vi "ControlUI_Main0.vi"(5 "Splash StatusRef":refnum<vi>, 7 "Splash VI Ref":refnum<vi>, 10 "Application":refnum<class "Application.lvclass">, 11 "Main.lvclass":refnum<class "Main.lvclass">) -> ()   [LabVIEW 2019, in "Main.lvclass"]
doc: "Developed by Kevin Thompson\nkevin@thompsonengineering.net\n\nCopyright 2018\nThompson Engineering, LLC"
uses:
  Main.lvclass
  <vilib>/TELLC/SMQ/Add States to Queue using MultiLine String with vData.vi
  Common/DataTypes/TD Async CmdMsg EventData--cluster.ctl
  DataTypes/Public Events--cluster.ctl
  DataTypes/Dependency--cluster.ctl
  DataTypes/Settings--cluster.ctl
  DataTypes/Control UI - AppData--cluster.ctl
  Log_Engine/Log_Engine.lvclass
  DAQ_Engine/DAQ_Engine.lvclass
  Config/Config.lvclass
  Application/Application.lvclass
  Application/DataTypes/AsynMsg_Application--enum.ctl
  Common/DataTypes/TD GetSet ActionSelect--enum.ctl
  Common/Startup/GBL System.vi
  DAQ_Engine/DataTypes/AsynCmd_DAQ_Engine--enum.ctl
  Common/DataTypes/Measurement Config--cluster.ctl
  Common/DataTypes/DAQState--enum.ctl
  Common/DataTypes/LogState--enum.ctl
  Common/DataTypes/TDMSState--enum.ctl
  Common/DataTypes/UpdateControlValue EvData--cluster.ctl
  DataTypes/DataProcessAuxData--cluster.ctl
  Common/DataTypes/DataProcAuxDat--Qref.ctl
  Common/DataTypes/ChannelWaveforms--cluster.ctl
  Common/DataTypes/InverterWaveforms--cluster.ctl
  Common/DataTypes/InverterWaveforms--QRef.ctl
  support/Data Algorithms/subvis/DataTypes/Gain control.ctl
  DataTypes/ProcessingState--enum.ctl
  DataTypes/ProcessingStateChg EvData--cluster.ctl
  DataTypes/InverterInfo--cluster.ctl
  DataTypes/ProcessInitParams--cluster.ctl
  DataTypes/StartProcInitParams--cluster.ctl
  <vilib>/TELLC/Dynamic CVT API/TD Dynamic CVT DVR--ref.ctl
  DataTypes/AsynMsg_Main--enum.ctl
  DataTypes/PrivateAsynEv_Main--enum.ctl
  Common/DataTypes/inverter info v2--cluster.ctl
  Common/DataTypes/inverter gain range--cluster.ctl
  Common/DataTypes/inverter offset range--cluster.ctl
  Common/DataTypes/Inverter database record v2--cluster.ctl
  support/Data Algorithms/subvis/DataTypes/ESR scaling--cluster.ctl
  <userlib>/_OpenG.lib/comparison/comparison.llb/String Changed__ogtk.vi
  <userlib>/_OpenG.lib/error/error.llb/Filter Error Codes (Array)__ogtk.vi
  Common/DataTypes/Acquisition Mode--cluster.ctl
panel:
  out "Next State":string
  in  "Trigger SelectInverter Event":bool
  in  "LeftPanelTab":T1(tab)=enum."Settings"
  out "InvSelLED":bool
  in  "Selected Inverter":string[](array[string])
  in  "SelectInverter":bool
  in  "Inverter List":i32[](listbox)
  in  "Settings.Signal scaling":T2[](array[typedef])
  in  "Samples RMS 9775":u32=3
  in  "Samples RMS 9215":u32=480000
  in  "Data Rate 9215 (S/s)":dbl=1200000.0 format="%#.6p"
  in  "Data Rate 9775(S/s)":dbl=3.0 format="%#.6p"
  out "DAQEnabled":bool=TRUE
  in  "DAQEnDis":bool
  out "LogEnabled":bool
  in  "LogEnDis":bool
  out "TDMSEnabled":bool
  in  "TDMSEnDis":bool
  in  "StopProcessing":bool caption="StopProcess"
  out "Processing":bool=TRUE
  in  "StartProcessing":bool caption="StartProcess"
  in  "UpdateDAQSettings":bool
  in  "Acqusition Mode":T3
  in  "cRIO Error\nReporting Mode":i32(ring) items=["DONTPRINT", "PRINTWARNINGS", "PRINTFATAL", "PRINTALL"]
  in  "MinCurrThreshold":dbl=1.5 caption="Minimum Current\nThreshold (A)" format="%.2f"
  in  "NumPF RdsToAvg":i32=2 caption="Number PF\nReads to Avg"
  in  "ESR alarm threshhold (%)":dbl=200.0
  in  "# readings to average":i32=40
  out "DP AuxData Size":i32
  out "InvWfmsQ DT size":i32
  in  "Inverter ID":string
  in  "toggle scrollbars":bool
  in  "toggle MainTabDbgPg":bool
  out "voltage fb":dbl caption="Voltage" format="%.3f"
  out "Current fb":dbl caption="Current" format="%.3f"
  out "Motor SP":dbl caption="Computed Motor\nPos Chg (in)" format="%.3f"
  out "In Range?":bool
  out "AVC Lockout":bool=TRUE
  out "Volts and Current Chart":T4(graph)
  out "VoltageError":dbl caption="Voltage Error" format="%.3f"
  in  "Launch_UI":bool caption="Launch UI"
  in  "Launch_UI 2":bool caption="Launch UI 2"
  in  "Launch_UI 3":bool caption="Launch UI 3"
  out "Current SP":dbl format="%.3f"
  in  "GraphEnable":bool
  out "Vsp_Sum":dbl format="%.2f"
  out "TotalVgain":dbl caption="Total Ctlr\nVgain" format="%.3f"
  out "DAQ Running":bool=TRUE
  out "MeasSet":T5={"Data Rate 9775"=3.0, "Data Rate 9215"=1200000.0, "Samples RMS 9215"=480000, "Samples RMS 9775"=3}
  out "DAQError":bool caption="DAQ Error"
  in  "SystemError":bool
  out "Sel_PowerFactor_Data":bool=TRUE
  in  "Show_PowerFactor_Data":bool
  out "Sel_TimeSeries_Data":bool
  in  "Show_TimeSeries_Data":bool
  out "Sel_ESR_Data":bool
  in  "Show_ESR_Data":bool
  in  "MainPanelTab":T6(tab)=enum."PowerFactorData"
  out "Max ESR":dbl format="%_4e"
  out "Inverter State":string
  out "Equivalent Series Resistance (ESR)":T7(graph)
  in  "StoreESR BLine":bool
  in  "UseSavedESR BLine":bool
  in  "set alarm":bool
  in  "reset averaging":bool
  in  "reset alarm":bool
  out "Inverter ESR status":bool
  out "Raw  ESR":dbl format="%.3e"
  out "Scaled & avgd ESR":dbl format="%_4e"
  in  "ESR scaling":T8[](array[typedef])
  out "Iout 60Hz":waveform(dbl)[](graph)
  out "Iout ripple":waveform(dbl)[](graph)
  out "Iin ripple":waveform(dbl)[](graph)
  out "DUT4 I-V":waveform(dbl)[](graph) caption="DUT 4"
  out "phase3 power data":T9 caption="Phase 1" {"Vout (RMS)" format="%0.2f"; "Iout (RMS)" format="%0.2f"; "PF" format="%.3g"}
  out "phase2 power data":T9 caption="Phase 1" {"Vout (RMS)" format="%0.2f"; "Iout (RMS)" format="%0.2f"; "PF" format="%.3g"}
  out "DUT3 I-V":waveform(dbl)[](graph) caption="DUT 3"
  out "DUT2 I-V":waveform(dbl)[](graph) caption="DUT 2"
  out "DUT1 I-V":waveform(dbl)[](graph) caption="DUT 1"
  out "phase1 power data":T9 caption="Phase 1" {"Vout (RMS)" format="%0.2f"; "Iout (RMS)" format="%0.2f"; "PF" format="%.3g"}
  in  "Dummy Vrms":dbl format="%.2g"
  in  "UseDummyVrms":bool
  out "phase4 power data":T9 caption="Phase 1" {"Vout (RMS)" format="%0.2f"; "Iout (RMS)" format="%0.2f"; "PF" format="%.3g"}
  in  "Page2Pg_button":bool
  in  "SettingsPg_button":bool
  in  "DataPg_button":bool
  in  "ConfigPg_button":bool
  in  "Exit":bool
  in  "TitleBar AppVerText":string="v2.0.2 build-003"
  in  "TitleBar Text":string="INVERTER   HEALTH   SCANNER   SYSTEM"
  in  "TitleBar":bool
  in  "StatusMsg":string caption="Status"
  in  "process sync":refnum<notifier>
  # "click to reset"
  # "UNUSED CONTROLS"
  # "Run Time Data Panel"
  # "Inverter Selection"
  # "right-click to open table editor"
  # "Configuration Panel"
  # "Settings Panel"
  # "cRIO  Settings"
  # "ESR Data"
  # "Time Series Data"
  # "DUT 1"
  # "DUT 2"
  # "DUT 3"
  # "DUT 4"
  # "Power Factor Data - Phase Current and Voltage"
  # "DUT 3"
  # "DUT 2"
  # "DUT 1"
  # "Current (A)"
  # "Voltage (V)"
  # "DUT 4"
  # "Debug Page"
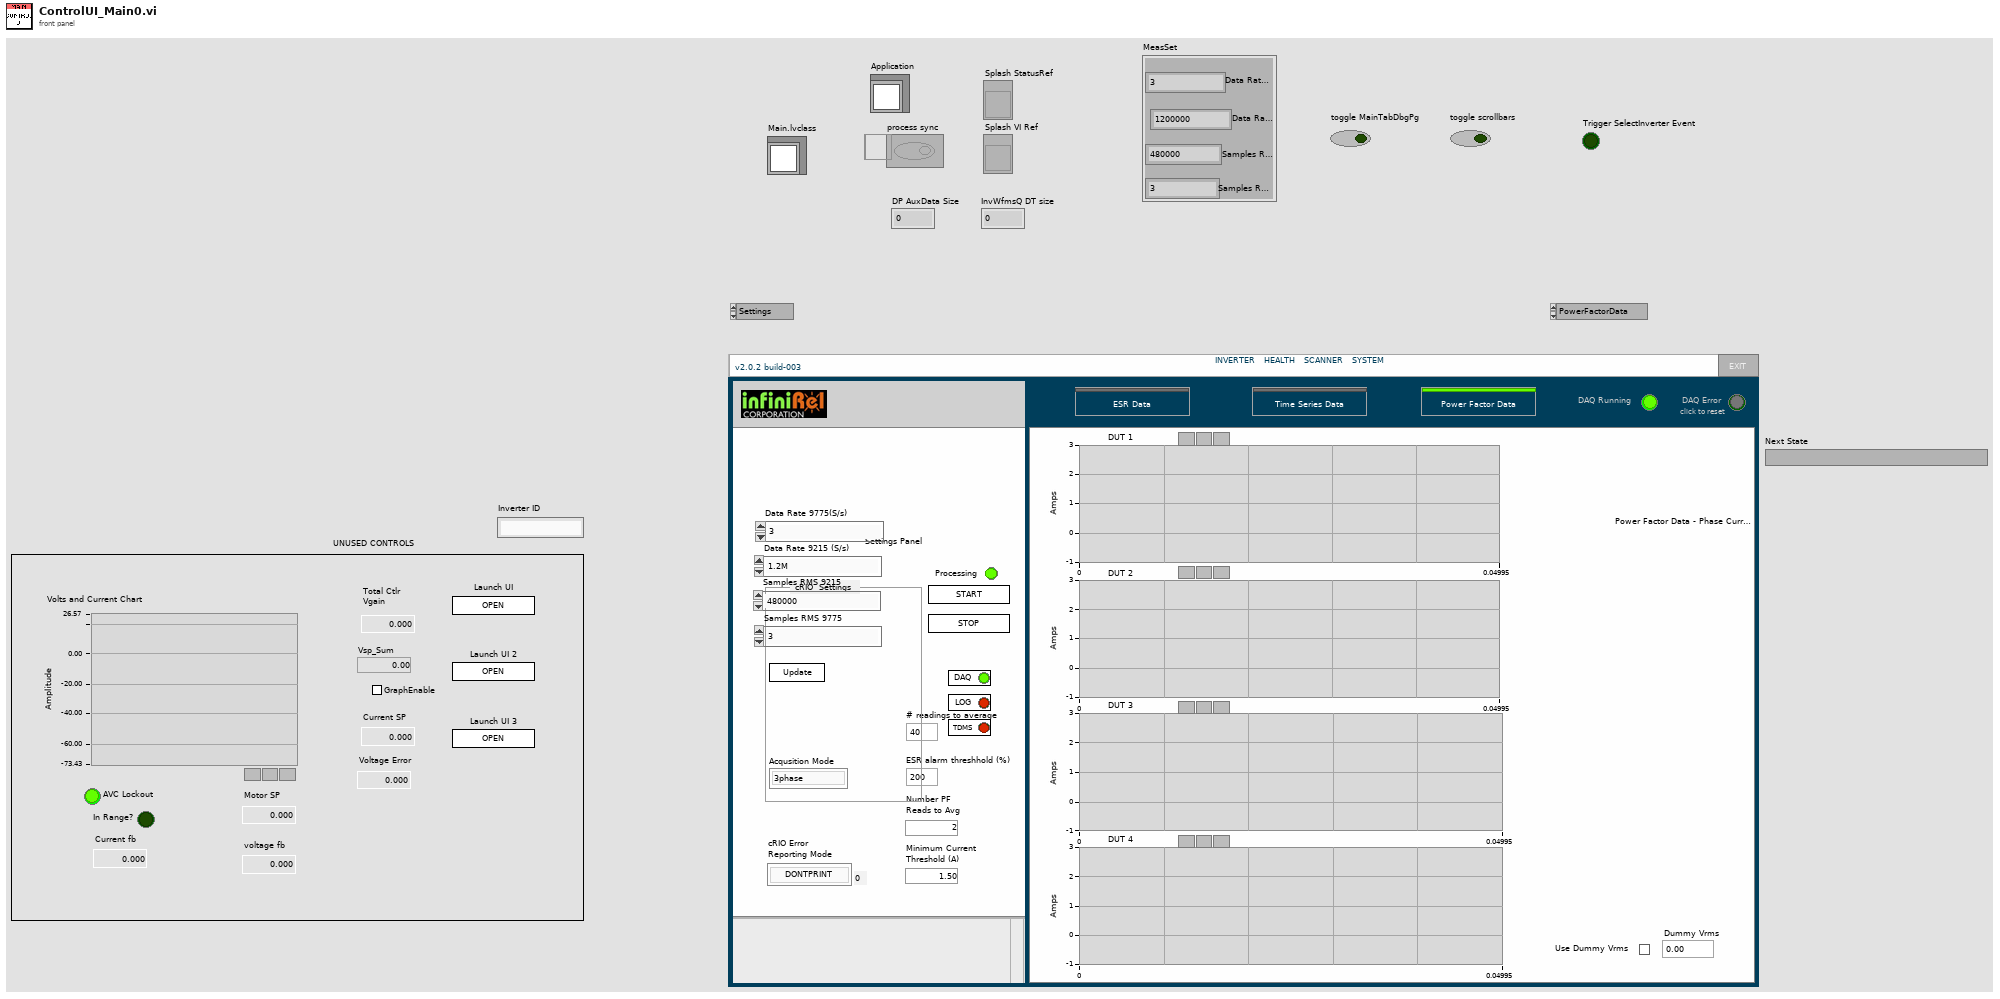
[diagram p1: front panel]
types:
  T1 = enum32{"Data", "InverterSel", "Config", "Settings"}
  T2 = typedef "Main.lvclass/Gain control.ctl" = cluster{"Iin ripple gain":dbl, "Iout ripple gain":dbl, "Iout 60Hz gain ":dbl, "Vout 60Hz gain ":dbl, "Iin ripple offest":dbl, "Iout ripple offset":dbl, "Iout 60Hz offset":dbl, "Vout 60Hz offset":dbl}
  T3 = typedef "Acquisition Mode--cluster.ctl" = enum16{"3phase", "Single"}
  T4 = cluster{"VoltageDyn":dbl, "CurrentDyn":dbl, "MotorV SP":dbl}
  T5 = typedef "Measurement Config--cluster.ctl" = cluster{"Data Rate 9775":dbl, "Data Rate 9215":dbl, "Samples RMS 9215":u32, "Samples RMS 9775":u32}
  T6 = enum32{"ESRData", "TimeSeriesData", "PowerFactorData", "DebugPage"}
  T7 = cluster{"ESR Baseline":dbl, "Alarm threshhold (%)":dbl, "Avg value":dbl}[]
  T8 = typedef "Main.lvclass/ESR scaling--cluster.ctl" = cluster{"Gain":dbl, "Offset":dbl}
  T9 = cluster{"PF":dbl, "Iout (RMS)":dbl, "Vout (RMS) ":dbl, "Power (W)":dbl}
  T10 = typedef "Main.lvclass/ProcessingState--enum.ctl" = enum16{"Idle", "Starting", "Running", "Done", "Error"}
  T11 = typedef "TD GetSet ActionSelect--enum.ctl" = enum16{"Init", "Get", "Set"}
  T12 = typedef "Main.lvclass/Control UI - AppData--cluster.ctl" = cluster{"Core":cluster{"Current VI Reference":refnum<vi>, "Close Panel on Exit?":bool}, "SMQ":refnum<queue>, "Initialized?":bool, "Self Reference":refnum<class "Main.lvclass">, "Simulation?":bool, "process sync":refnum<notifier>, "vData":variant, "Settings":T13, "Dependency":T14, "Public Events":T15, "Splash StatusRef":refnum<vi>, "Splash VI Ref":refnum<vi>, "RunTimeSystem?":bool, "StatusMsg Ref":refnum<vi>, "AppTerminateEv":refnum<user-event>, "MenuRef":refnum<k9>, "DAQEnabled":bool, "LoggingEnabled":bool, "TDMS Enabled":bool, "Application":refnum<class "Application.lvclass">, "InvWfmsQ-DT":T16, "DPAuxDataQ":T17, "ProcessingState":T10, "DisplayLoopInterval":u32, "MenuBarShown?":bool, "InverterNames[]":string[], "InverterLUT Dict":T18}
  T13 = typedef "Main.lvclass/Settings--cluster.ctl" = cluster{"Simulation":bool, "Signal scaling":T2[], "ESR scaling":T8[], "num readings to average":i32[], "ESR alarm threshhold (%)":i32[], "UseDummyVrms":bool, "Dummy Vrms":dbl, "Inverter Database File":path, "default Inverter (name)":string[]}
  T14 = typedef "Main.lvclass/Dependency--cluster.ctl" = cluster{"Config":refnum<class "Config.lvclass">, "DAQ":refnum<class "DAQ_Engine.lvclass">, "Log_Engine":refnum<class "Log_Engine.lvclass">}
  T15 = typedef "Main.lvclass/Public Events--cluster.ctl" = cluster{"Main.AsyncCmd Event":refnum<user-event>, "Main.AsyncMsg Event":refnum<user-event>, "stop process":refnum<user-event>, "UpdateControlValue Ev":refnum<user-event>, "ProcessingStateChg Ev":refnum<user-event>}
  T16 = typedef "InverterWaveforms--QRef.ctl" = refnum<queue>
  T17 = typedef "DataProcAuxDat--Qref.ctl" = refnum<queue>
  T18 = typedef "TD Dynamic CVT DVR--ref.ctl" = refnum<data-value>
  T19 = cluster{"AvgPF":dbl, "IoutRMS_A":dbl, "VoutRMS_V":dbl, "Power_W":dbl}
  T20 = typedef "DataProcessAuxData--cluster.ctl" = cluster{"Time Stamp":timestamp, "Raw ESR sum":dbl, "Inv 1 ON?":bool, "Average scaled ESR sum":dbl, "Inv 1 over threshold?":bool, "Inv 1 ESR":cluster{"ESR Baseline":dbl, "Alarm threshhold (%)":dbl, "Avg value":dbl}, "Max ESR":dbl}
  T21 = cluster{"ESR Baseline":dbl, "Alarm threshhold (%)":dbl, "Avg value":dbl}
  T22 = typedef "InverterWaveforms--cluster.ctl" = T23[]
  T23 = typedef "ChannelWaveforms--cluster.ctl" = cluster{"Iin ripple ":waveform(dbl), "Iout ripple ":waveform(dbl), "Iout 60Hz":waveform(dbl), "Vout 60Hz":waveform(dbl)}
  T24 = typedef "DAQ_Engine.lvclass/AsynCmd_DAQ_Engine--enum.ctl" = enum16{"DAQ.EnableDAQ", "DAQ.ClearDAQError", "DAQ.SetMeasConfig", "DAQ.SetAcqMode", "DAQ.SetErrorReporting"}
  T25 = typedef "Main.lvclass/StartProcInitParams--cluster.ctl" = cluster{"InverterInfo":T26, "ProcessInitParams":T27}
  T26 = typedef "InverterInfo--cluster.ctl" = cluster{"Inverter ID":string}
  T27 = typedef "Main.lvclass/ProcessInitParams--cluster.ctl" = cluster{"MinCurrThreshold":dbl, "NumPF RdsToAvg":i32, "ESR alarm threshhold (%)":dbl, "# readings to average":i32}
  T28 = typedef "Main.lvclass/PrivateAsynEv_Main--enum.ctl" = enum16{"PrivMain.UpdateMeasSettings", "PrivMain.UpdateAcqMode", "PrivMain.UpdateDAQState", "PrivMain.UpdateLogState", "PrivMain.UpdateTDMSState", "PrivMain.UpdateProcessingState", "PrivMain.Stop&Terminate", "PrivMain.CurrInverterUpdated", "PrivMain.UpdateStoreUseESRBaseline", "PrivMain.SetUnsetAlarm&ESRBLine", "PrivMain.ResetAveraging"}
  T29 = typedef "Main.lvclass/AsynMsg_Main--enum.ctl" = enum16{"Main.CurrInverterUpdated"}
  T30 = typedef "DAQState--enum.ctl" = enum16{"Unknown", "Stopped", "Running", "Error"}
  T31 = cluster{"VoltageDyn":dbl, "CurrentDyn":dbl, "MotorV SP":dbl}[]
  T32 = enum32{"invalid app kind", "Development System", "Run Time System", "Student Edition", "Embedded LabVIEW", "Evaluation", "Custom"}
  T33 = typedef "Application.lvclass/AsynMsg_Application--enum.ctl" = enum16{"Application.AppClassReference"}
  T34 = enum16{"Left Button", "Center Button", "Right Button", "Window Close"}
  T35 = enum32{"Invalid", "Standard", "Closed", "Hidden", "Minimized", "Maximized"}
  T36 = enum32{"Invalid", "Default", "Floating", "Floating/Auto-Hide", "Modal"}
  T37 = typedef "Inverter database record v2--cluster.ctl" = cluster{"name":string, "last updated":timestamp, "type":string, "inverter Info":T38, "gain range":T39, "offset range":T40, "gain actual":dbl, "offset actual":dbl, "power level":dbl, "minimum current":dbl, "resistance single phase":dbl, "resistance 3 phase":dbl, "set flag":u16}
  T38 = typedef "inverter info v2--cluster.ctl" = cluster{"manufacturer":string, "model":string, "product":string, "serial":string, "power class":string, "year manf":string}
  T39 = typedef "inverter gain range--cluster.ctl" = cluster{"gain max":dbl, "gain min":dbl, "gain increment":dbl}
  T40 = typedef "inverter offset range--cluster.ctl" = cluster{"offset max":dbl, "offset min":dbl, "offset increment":dbl}
  T41 = typedef "Application.lvclass/AVC2_TouchScreen_MainUI - AppData--cluster.ctl" = cluster{"Core":cluster{"Current VI Reference":refnum<vi>, "Close Panel on Exit?":bool}, "SMQ":refnum<queue>, "Initialized?":bool, "Public Events":T42, "Dependency":T43, "MenuRef":refnum<k9>, "RuntimeSystem?":bool, "StatusMsg Ref":refnum<vi>, "PrevSeqFolder":path, "SeqRunning?":bool, "SeqExecStatus":T44, "SeqAborted?":bool, "LoadSeqStatus":T45, "Session Settings":T46, "SessionSettings Set?":bool, "DAQEnabled":bool, "LoggingEnabled":bool, "TDMS Enabled":bool, "Logger State Data":T47, "Splash VI Ref":refnum<vi>, "Splash StatusRef":refnum<vi>, "Motor_LA CtrlUI VI Ref":refnum<vi>, "Dflt_Motor_LA Vel":dbl, "Motor_TT CtrlUI VI Ref":refnum<vi>, "Dflt_Motor_TT Vel":dbl, "App Settings":T49, "ExpSubsysRsp":string, "ExpSubsysRspTime":dbl, "Motor_Osc CtrlUI VI Ref":refnum<vi>, "Dflt_Motor_Osc Vel":dbl, "RGrph":refnum<queue>, "Private Events":T59, "WeldGrph":refnum<queue>, "SeqStartTime (s)":dbl, "XYGraphPlotData":T60, "Seq WeldProfileData":cluster{"Time (s)":dbl[], "WeldCurrent":dbl[]}, "Rect":T61, "MenuBarShown?":bool, "Disable Oscillator Motor":bool, "PurgeTimerExp":dbl, "vData":variant, "WELD COUNT":i32}
  T42 = typedef "Application.lvclass/Public Events--cluster.ctl" = cluster{"Application.AsyncCmd Event":refnum<user-event>, "Application.AsyncMsg Event":refnum<user-event>, "stop process":refnum<user-event>, "Application.ControlStateChg Event":refnum<user-event>, "Application.RadialGraph Event":refnum<user-event>}
  T43 = typedef "Application.lvclass/Dependency--cluster.ctl" = cluster{"Config":refnum<class "Config.lvclass">, "DAQ":refnum<class "DAQ.lvclass">, "Sequencer":refnum<class "Sequencer.lvclass">, "LogEngine":refnum<class "LogEngine.lvclass">, "ErrorHandler":refnum<class "ErrorHandler.lvclass">, "DataQueues":refnum<class "DataQueues.lvclass">, "Motion":refnum<class "Motion.lvclass">, "PID_Ctlr":refnum<class "PID_Ctlr.lvclass">, "Welder":refnum<class "Welder.lvclass">}
  T44 = typedef "Sequencer.lvclass/SeqExecStatus--enum.ctl" = enum16{"Unknown", "Idle", "Running", "Aborted"}
  T45 = typedef "Sequencer.lvclass/LoadSeqStatus--enum.ctl" = enum16{"Unknown", "InProgress", "Loaded", "Failed"}
  T46 = typedef "SessionSettings--cluster.ctl" = cluster{"Job_ID":string, "Operator_ID":string, "Station_ID":string, "Job_Description":string}
  T47 = typedef "LogEngine.lvclass/TD Logger State Data--cluster.ctl" = cluster{"Logger State":T48, "TDMS Logging State":T48, "LogFile path":path, "TDMS File path":path, "vData":variant}
  T48 = typedef "LogEngine.lvclass/TD Logger State--enum.ctl" = enum16{"Unknown", "Logging", "NotLogging", "Error"}
  T49 = typedef "Application.lvclass/Settings--cluster.ctl" = cluster{"Placeholder":bool, "ProfilePlotScaleFactor":dbl, "ConversionFactors":T50, "SystemDefaults":T51, "TimingIntervals":T52, "AO IONames":T53, "DO IONames":T54, "UI Labels":T55, "AI IONames":T56, "DI IONames":T57, "TurntableType":T58, "Torch IncrButton displ (in)":dbl, "preventSimulatedEMOAbort":bool}
  T50 = typedef "Application.lvclass/ConversionFactors--cluster.ctl" = cluster{"WeldCurrentSP I/V":dbl, "Turntable RPM/V":dbl, "VoltageDynFB V/V":dbl, "CurrentDynFB I/V":dbl}
  T51 = typedef "Application.lvclass/SystemDefaults--cluster.ctl" = cluster{"AVCLockout":dbl, "TurntableJog":dbl, "ProfilePlotScaleFactor":dbl, "DefaultSeqFile":string, "defaultVelocitySP":dbl}
  T52 = typedef "Application.lvclass/Timing Intervals--cluster.ctl" = cluster{"DAQDisplay Interval":i32, "DAQRd&MtrSP Interval":u32, "WriteLogFile Interval":u32, "SeqHoldLoop Interval":u32, "SeqRampLoop Interval":u32, "ArcEnRelayToggle Interval":u32}
  T53 = typedef "AO IONames--cluster.ctl" = cluster{"Weld Current":string, "Turntable Speed":string, "Turntable Jog":string}
  T54 = typedef "DO IONames--cluster.ctl" = cluster{"Arc Enable Relay":string, "AVC Lockout Relay":string, "Turntable Enable Relay":string, "Turntable Jog Switch":string}
  T55 = typedef "UI Controls-Indicators Labels--cluster.ctl" = cluster{"SeqRunning":string, "Process Complete":string, "AVC Lockout":string, "Step Comment":string, "StepCntDn":string, "SeqList":string, "Current SP":string, "VspOffset":string, "WeldCurrentWfmChart":string, "Turntable En (Anlg)":string}
  T56 = typedef "AI IONames--cluster.ctl" = cluster{"AI TaskName":string, "VoltageDyn":string, "CurrentDyn":string}
  T57 = typedef "DI IONames--cluster.ctl" = cluster{"DI TaskName":string, "EMO_Signal":string}
  T58 = typedef "TurntableType--enum.ctl" = enum16{"SmartMotor", "Analog"}
  T59 = typedef "Application.lvclass/Private Events--cluster.ctl" = cluster{"Private.AsyncCmd Event":refnum<user-event>, "Private.AsyncMsg Event":refnum<user-event>}
  T60 = typedef "Application.lvclass/WeldCurrent_GraphPlotData--cluster.ctl" = cluster{"Timeoffset(s)":dbl[], "WeldCurrent[]":dbl[]}
  T61 = typedef "LVRectTypeDef.ctl" = cluster{"Left":i16, "Top":i16, "Right":i16, "Bottom":i16}
  T62 = typedef "Main.lvclass/AsynCmd_Main--enum.ctl" = enum16{"Main.StartProcessing", "Main.StopProcessing", "Main.RefreshInverterList"}
  T63 = typedef "DAQ_Engine.lvclass/DAQStateEvData--cluster.ctl" = cluster{"DAQState":T30, "vData":variant}
  T64 = typedef "LogState--enum.ctl" = enum16{"Unknown", "Stopped", "Running", "Error"}
  T65 = typedef "Log_Engine.lvclass/LogStateEvData--cluster.ctl" = cluster{"LogState":T64, "vData":variant}
  T66 = typedef "TDMSState--enum.ctl" = enum16{"Unknown", "Stopped", "Running", "Error"}
  T67 = typedef "Log_Engine.lvclass/TDMSStateEvData--cluster.ctl" = cluster{"TDMSState":T66, "vData":variant}
  T68 = typedef "DAQ_Engine.lvclass/Public Events--cluster.ctl" = cluster{"DAQ_Engine.AsyncCmd Event":refnum<user-event>, "DAQ_Engine.AsyncMsg Event":refnum<user-event>, "stop process":refnum<user-event>, "DAQ_Engine.DAQStateChg Ev":refnum<user-event>, "DAQ_Engine.MeasSettingsChg Ev":refnum<user-event>, "DAQ_Engine.AcqModeChg Ev":refnum<user-event>}
  T69 = typedef "Log_Engine.lvclass/Public Events--cluster.ctl" = cluster{"Log_Engine.AsyncCmd Event":refnum<user-event>, "Log_Engine.AsyncMsg Event":refnum<user-event>, "stop process":refnum<user-event>, "Log_Engine.LogStateChg Ev":refnum<user-event>, "Log_Engine.TDMSStateChg Ev":refnum<user-event>}
  T70 = cluster{"Current VI Reference":refnum<vi>, "Close Panel on Exit?":bool}
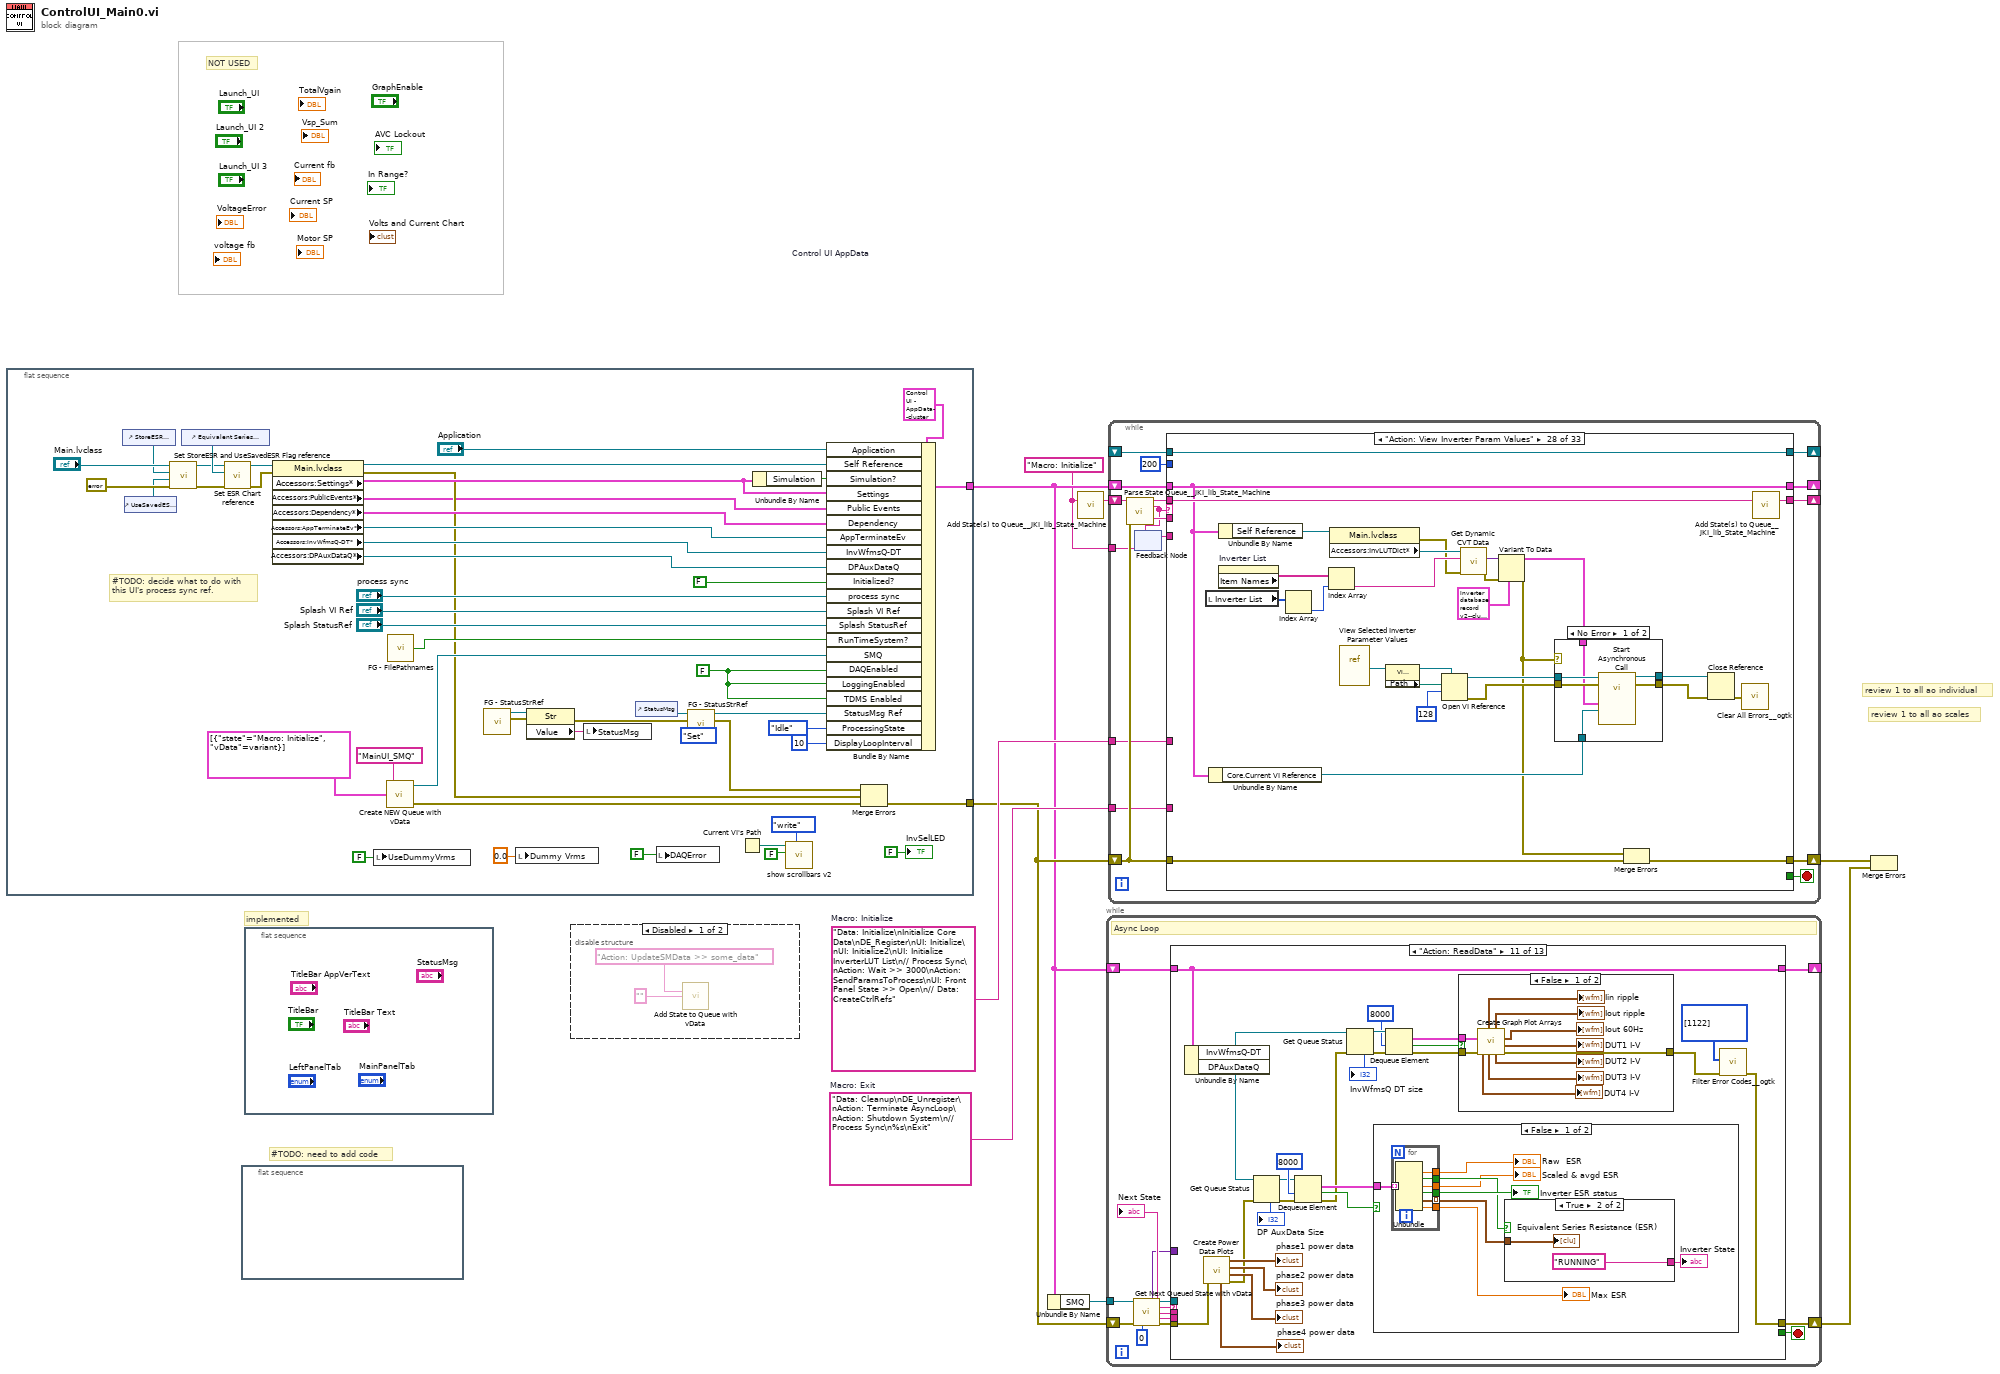
[diagram p0: block diagram]
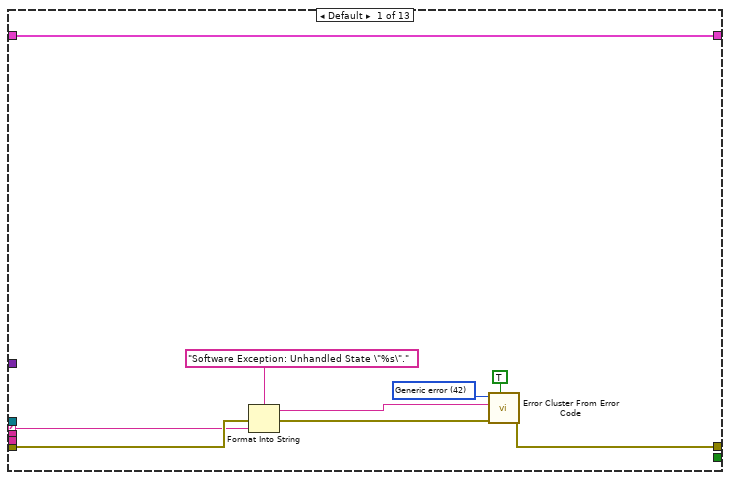
[diagram p3: hidden frame]
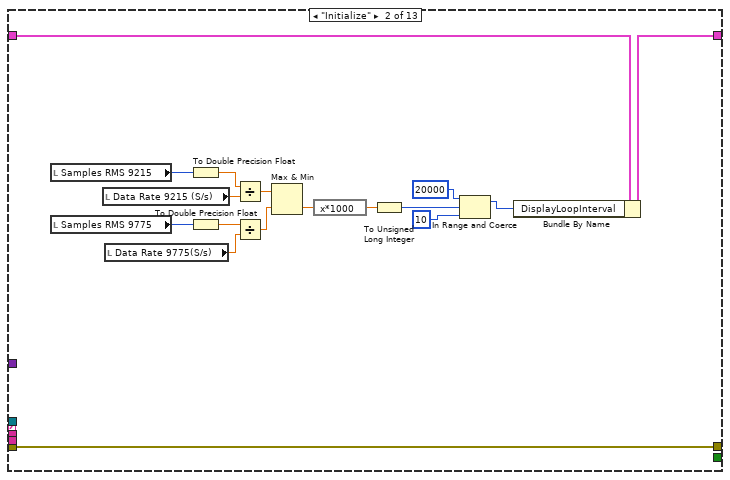
[diagram p4: hidden frame]
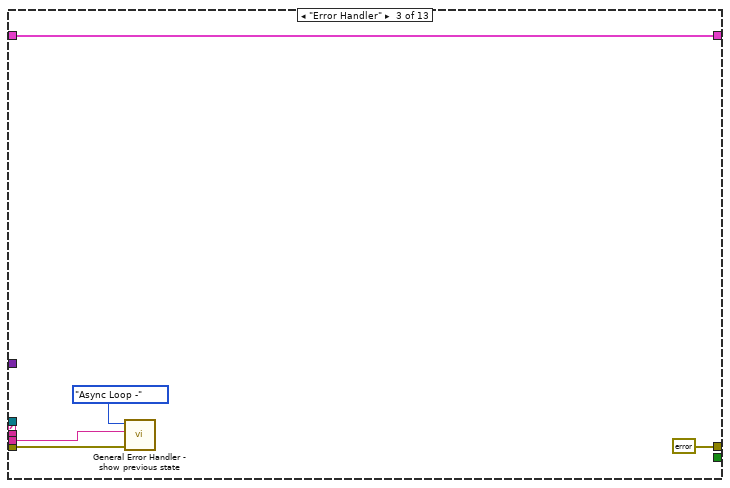
[diagram p5: hidden frame]
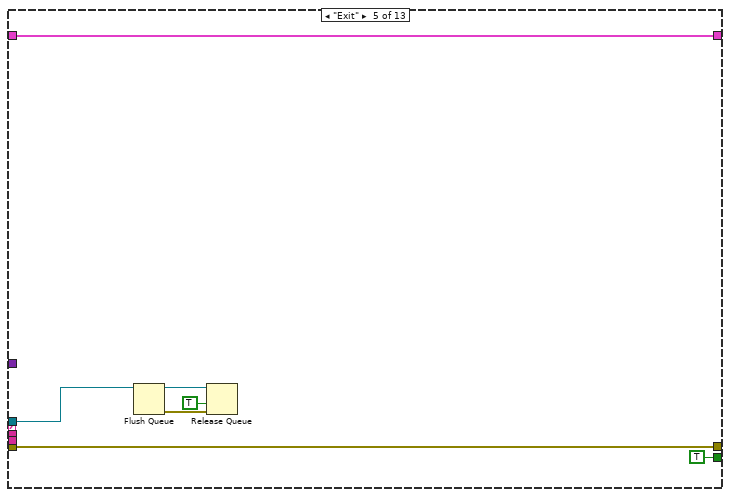
[diagram p7: hidden frame]
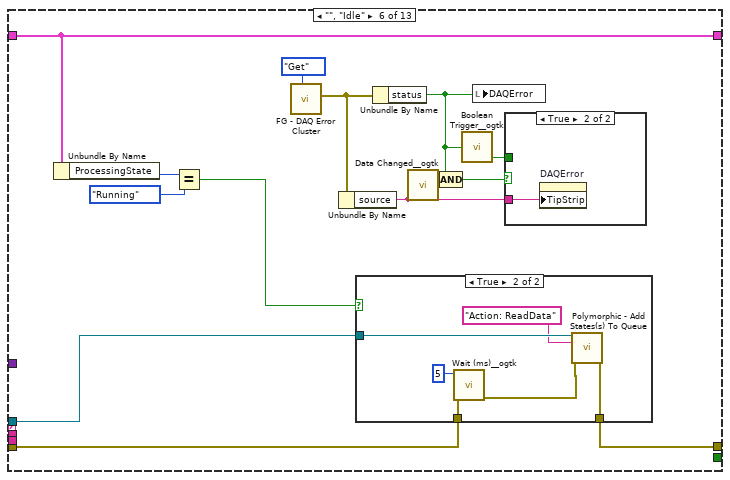
[diagram p8: hidden frame]
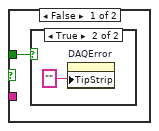
[diagram p9: hidden frame]
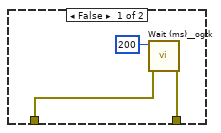
[diagram p11: hidden frame]
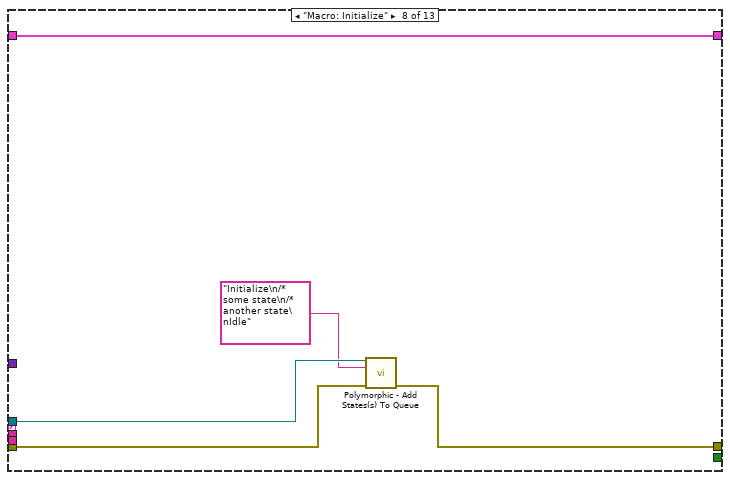
[diagram p13: hidden frame]
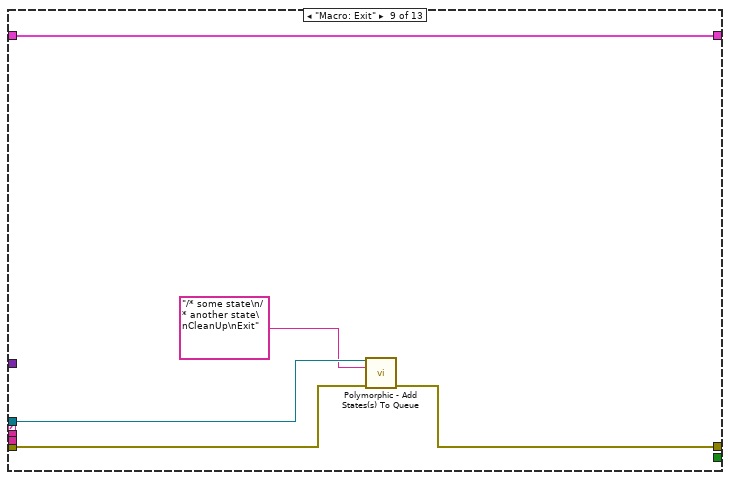
[diagram p14: hidden frame]
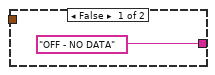
[diagram p16: hidden frame]
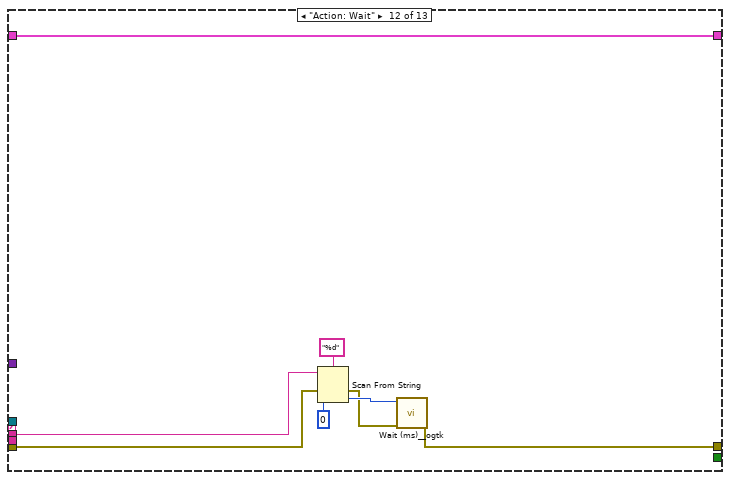
[diagram p19: hidden frame]
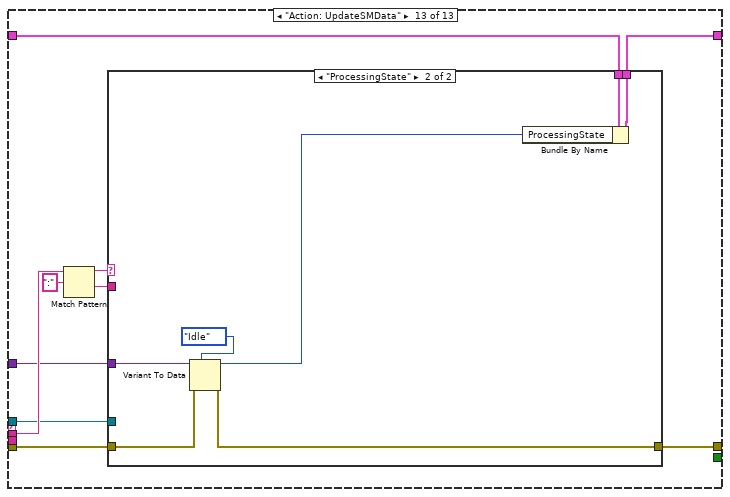
[diagram p20: hidden frame]
diagram:
  w7 = "Data: Cleanup\nDE_Unregister\nAction: Terminate AsyncLoop\nAction: Shutdown System\n// Process Sync\n%s\nExit"  # Macro: Exit
  w8 = "Data: Initialize\nInitialize Core Data\nDE_Register\nUI: Initialize\nUI: Initialize2\nUI: Initialize InverterLUT List\n// Process Sync\nAction: Wait >> 3000\nAction: SendParamsToProcess\nUI: Front Panel State >> Open\n// Data: CreateCtrlRefs"  # Macro: Initialize
  w1 = "Macro: Initialize"
  # "review 1 to all ao scales"
  # "review 1 to all ao individual"
  # "implemented"
  # "#TODO: need to add code"
  # "NOT USED"
  n1 = flat-sequence {
    tunnel: [w58] -> w4
    tunnel: [w43] -> w6
    frame #0 {
      w29 = FALSE
      w50 = T12 {"Core"={"Current VI Reference"=refnum, "Close Panel on Exit?"=FALSE}, "SMQ"=refnum, "Initialized?"=FALSE, "Self Reference"=refnum, "Simulation?"=FALSE, "process sync"=refnum, "vData"=variant, "Settings"={"Simulation"=FALSE, "Signal scaling"=[], "ESR scaling"=[], "num readings to average"=[], "ESR alarm threshhold (%)"=[], "UseDummyVrms"=FALSE, "Dummy Vrms"=0.0, "Inverter Database File"=path "", "default Inverter (name)"=[]}, "Dependency"={"Config"=refnum, "DAQ"=refnum, "Log_Engine"=refnum}, "Public Events"={"Main.AsyncCmd Event"=refnum, "Main.AsyncMsg Event"=refnum, "stop process"=refnum, "UpdateControlValue Ev"=refnum, "ProcessingStateChg Ev"=refnum}, "Splash StatusRef"=refnum, "Splash VI Ref"=refnum, "RunTimeSystem?"=FALSE, "StatusMsg Ref"=refnum, "AppTerminateEv"=refnum, "MenuRef"=refnum, "DAQEnabled"=FALSE, "LoggingEnabled"=FALSE, "TDMS Enabled"=FALSE, "Application"=refnum, "InvWfmsQ-DT"=refnum, "DPAuxDataQ"=refnum, "ProcessingState"=enum."Idle", "DisplayLoopInterval"=0, "MenuBarShown?"=FALSE, "InverterNames[]"=[], "InverterLUT Dict"=refnum}  # Control UI AppData
      # "#TODO: decide what to do with\nthis UI's process sync ref."
      n2 = control-ref of="StoreESR BLine"() -> (w10:refnum<vi>)
      n3 = control-ref of="UseSavedESR BLine"() -> (w11:refnum<vi>)
      n4 = call "Set StoreESR and UseSavedESR Flag reference.vi"("error in (no error)"=errorcluster {"status"=FALSE, "code"=0, "source"=""} ("error constant"), "UseSavedESR BLine Ref"=w11, "StoreESR BLine Ref"=w10, "Main in"="Main.lvclass") -> ("error out"=w14:errorcluster, "Main out"=w15:refnum<class "Main.lvclass">)  [unwired: 6 in]
      n5 = control-ref of="Equivalent Series Resistance (ESR)"() -> (w17:refnum<vi>)
      n6 = call "Set ESR Chart reference.vi"("error in (no error)"=w14, "ESR Chart Ref"=w17, "Main in"=w15) -> ("error out"=w12:errorcluster, "Main out"=w18:refnum<class "Main.lvclass">)  [unwired: 7 in]
      n7 = property class="Main.lvclass"(reference=w18, error in=w12) -> (reference out=w21:refnum<class "Main.lvclass">, error out=w22:errorcluster, "Accessors:Settings*"=w52:T13, "Accessors:PublicEvents*"=w20:T15, "Accessors:Dependency*"=w54:T14, "Accessors:AppTerminateEv*"=w49:refnum<user-event>, "Accessors:InvWfmsQ-DT*"=w28:T16, "Accessors:DPAuxDataQ*"=w27:T17)
      n8 = local write "UseDummyVrms"(FALSE ("UseDummyVrms")) -> ()
      n9 = call <vilib>:"Create NEW Queue with vData.vi"("Initial States"=cluster{"state":string, "vData":variant}[] [{"state"="Macro: Initialize", "vData"=variant}], "Name (SMQ)"="MainUI_SMQ") -> ("error out"=w44:errorcluster, "queue out"=w48:refnum<queue>)  [unwired: 2 in]
      n10 = call "FG - FilePathnames.vi"() -> ("RunTimeSys?"=w45:bool)  [unwired: 4 in, 1 out]
      n11 = call "FG - StatusStrRef.vi"() -> ("StatusStr Ref out"=w42:refnum<vi>, "error out"=w41:errorcluster)  [unwired: 9 in]
      n12 = local write "Dummy Vrms"(0.0 ("Dummy Vrms")) -> ()
      n13 = property class="Str"(reference=w42, error in=w41) -> (error out=w40:errorcluster, "Value"=w39:string)  [unwired: 1 out]
      n14 = local write "StatusMsg"(w39) -> ()
      n15 = control-ref of="StatusMsg"() -> (w38:refnum<vi>)
      n16 = local write "DAQError"(FALSE ("SystemError")) -> ()
      n17 = call "FG - StatusStrRef.vi"("StatusStr Ref in"=w38, "error in (no error)"=w40, "action (Get)"=TD_GetSet_ActionSelect--enum."Set") -> ("StatusStr Ref out"=w36:refnum<vi>, "error out"=w35:errorcluster)  [unwired: 6 in]
      n18 = Current VI's Path() -> (path=w34:path)
      n19 = Unbundle By Name(w52) -> ("Simulation"=w53:bool)
      n20 = call <vilib>:"show scrollbars v2.vi"("mode (read)"=enum16{"read", "write", "toggle"}."write", "ShowScrollbars?"=FALSE, "vi path"=w34) -> ()  [unwired: 4 in, 2 out]
      n21 = Bundle By Name(cluster=w50, "Application"="Application", "Self Reference"=w21, "Simulation?"=w53, "Settings"=w52, "Public Events"=w20, "Dependency"=w54, "AppTerminateEv"=w49, "InvWfmsQ-DT"=w28, "DPAuxDataQ"=w27, "Initialized?"=FALSE, "process sync"="process sync", "Splash VI Ref"="Splash VI Ref", "Splash StatusRef"="Splash StatusRef", "RunTimeSystem?"=w45, "SMQ"=w48, "DAQEnabled"=w29, "LoggingEnabled"=w29, "TDMS Enabled"=w29, "StatusMsg Ref"=w36, "ProcessingState"=ProcessingState--enum."Idle", "DisplayLoopInterval"=u32 10) -> (w58:T12)
      n22 = Merge Errors(w35, w22, w44) -> (w43:errorcluster)
      "InvSelLED" <- FALSE ("InvSelLED")
    }
  }
  n23 = flat-sequence {
    frame #0 {
    }
  }
  n24 = flat-sequence {
    frame #0 {
    }
  }
  n25 = disable-structure shown="Disabled" {
    frame Disabled {
      n26 = call <vilib>:"Add State to Queue with vData.vi"("state in"="Action: UpdateSMData >> some_data", "vData (\"\")"="") -> ()  [unwired: 10 in, 4 out]
    }
    frame Enabled {
    }
  }
  n27 = Unbundle By Name(w4) -> ("SMQ"=w5:refnum<queue>)
  n28 = call <vilib>:"Add State(s) to Queue__JKI_lib_State_Machine.vi"("State(s) in (\"\")"=w1) -> ("States Out"=w9:string)  [unwired: 14 in]
  n29 = while {
    shift-right: [w70] -> w2
    shift-left: w6 -> [w72]
    tunnel: w5 -> [w68]
    shift-right: [w66] -> _
    shift-left: w4 -> [w67]
    stop <- w61 stop-if-true
    # "Async Loop"
    n30 = call <vilib>:"Get Next Queued State with vData.vi"("queue in"=w68, "error in (no error)"=w72, "timeout (100)"=0) -> ("vData out"=w65:variant, "queue out"=w69:refnum<queue>, "Next State"=w73:string, "queued msg"=w63:string, "Prev State"=w62:string, "error out"=w71:errorcluster)  [unwired: 6 in, 1 out]
    "Next State" <- w73
    n31 = case shown="\"Action: ReadData\"" w73 {
      tunnel: w69 -> [_ _ _ _ w107 w126 _ w145 w150 _ _ _ w222]
      tunnel: w63 -> [_ _ _ _ _ _ _ _ _ _ _ w211 w224]
      selector: w73 -> [w74 _ _ _ _ _ _ _ _ _ _ _ _]
      tunnel: w71 -> [w76 w99 w101 w106 w113 w124 w141 w144 w149 w153 w172 w210 w219]
      tunnel: [w75 w99 errorcluster {"status"=FALSE, "code"=0, "source"=""} ("error constant") w106 w113 w127 w141 w143 w148 w153 w156 w213 w218] -> w70
      tunnel: w67 -> [w82 w97 w104 w105 w112 w125 w140 w146 w151 w152 w179 w216 w221]
      tunnel: [w82 w98 w104 w105 w112 w125 w140 w146 w151 w152 w179 w216 w220] -> w66
      tunnel: w65 -> [_ _ _ _ _ _ _ _ _ _ _ _ w223]
      tunnel: w62 -> [_ _ w100 _ _ _ _ _ _ _ _ _ _]
      tunnel: [_ _ _ _ TRUE _ _ _ _ _ _ _ _] -> w61
      frame Default {
        w78 = 42 items=["No error", "Argument error", "Memory is full", "Out of zone", "End of file", "File already open", "Generic file I/O error", "File not found", "File permission error", "Disk is full", "Duplicate path", "Too many files open", "System feature not enabled", "Resource file not found", "Cannot add resource", "Resource not found", "Image not found", "Image memory error", "Pen does not exist", "Config type invalid", "Config token not found", "Config parse error", "Config memory error", "Bad external code format", "Bad external code offset", "External code not present", "Null window", "Destroy window error", "Null menu", "Print aborted", "Bad print record", "Print driver error", "Windows error during printing", "Memory error during printing", "Print dialog error", "Generic print error", "Invalid device refnum", "Device not found", "Device parameter error", "Device unit error", "Cannot open device", "Device call aborted", "Generic error", "Cancelled by user", "Object ID too low", "Object ID too high", "Object not in heap", "Unknown heap", "Unknown object (invalid DefProc)", "Unknown object (DefProc not in table)", "Message out of range", "Invalid (null) method", "Unknown message", "Manager call not supported", "Bad address", "Network operation in progress", "Network operation timed out", "Connection is busy", "Network attribute not supported", "Network error", "Address in use", "System out of memory", "Connection aborted", "Connection refused", "Not connected", "Already connected", "Connection closed", "Initialization error (interapplication manager)", "Bad occurrence", "Wait on unbound occurrence handler", "Occurrence queue overflow", "Datalog type conflict", "Unused", "Unrecognized type (interapplication manager)", "Memory corrupt", "Failed to make temporary DLL", "Old CIN version", "Drag socket not found", "Failed to load drop-object", "Failed to register OLE object", "Failed to release OLE object", "Format specifier type mismatch", "Unknown format specifier", "Too few format specifiers", "Too many format specifiers", "Scan failed", "Newer CIN version", "Error converting to variant", "Runtime menu error", "Password tampered", "Variant attribute not found", "Incompatible variant data type", "Event data is not available", "Event Store is not present", "Occurrence is not found", "Event Queue is not created", "Event info is not available", "Refnum passed is NULL", "Error retrieving Class GUID", "Error retrieving CoClass GUID", "Error retrieving TypeLib GUID.", "Bad built application magic bytes.", "Specific driver is different from the specific driver associated with the Logical Name.", "There is no session opened to the class driver.", "Max Error", "MAX - Error with config objects", "MAX - Error loading configuration", "MAX - Group not supported"]
        n32 = Format Into String(format string="Software Exception: Unhandled State \"%s\"." ("message"), error in=w76, w74) -> (resulting string=w79:string, error out=w80:errorcluster)  [unwired: 1 in]
        n33 = call <vilib>:"Error Cluster From Error Code.vi"("show call chain? (False)"=TRUE, "error in (no error)"=w80, "error message (\"\")"=w79, "error code (0)"=w78) -> ("error out"=w75:errorcluster)  [unwired: 5 in]
      }
      frame "Initialize" {
        n34 = local read "Samples RMS 9215"() -> (w92:u32)
        n35 = local read "Samples RMS 9775"() -> (w91:u32)
        n36 = local read "Data Rate 9215 (S/s)"() -> (w93:dbl)
        n37 = local read "Data Rate 9775(S/s)"() -> (w90:dbl)
        n38 = To Double Precision Float(number=w92) -> (double precision float=w96:dbl)
        n39 = To Double Precision Float(number=w91) -> (double precision float=w89:dbl)
        n40 = Divide(x=w96, y=w93) -> (x/y=w88:dbl)
        n41 = Divide(x=w89, y=w90) -> (x/y=w87:dbl)
        n42 = Max & Min(x=w88, y=w87) -> (min(x,y)=w86:dbl)  [unwired: 1 out]
        n43 = expression code="x*1000"(w86) -> (w95:dbl)
        n44 = To Unsigned Long Integer(number=w95) -> (unsigned 32bit integer=w94:u32)
        n45 = In Range and Coerce(upper limit=u32 20000, x=w94, lower limit=u32 10) -> (coerced(x)=w83:u32)  [unwired: 1 out]
        n46 = Bundle By Name(cluster=w97, "DisplayLoopInterval"=w83) -> (w98:T12)
      }
      frame "Error Handler" {
        n47 = call "General Error Handler - show previous state.vi"("error in (no error)"=w101, "Previous State"=w100, "Loop Select"=enum16{"Event Loop -", "Async Loop -"}."Async Loop -") -> ()  [unwired: 7 in, 2 out]
      }
      frame "CleanUp" {
      }
      frame "Exit" {
        n48 = Flush Queue(queue=w107) -> (queue out=w110:refnum<queue>, error out=w109:errorcluster)  [unwired: 1 in, 1 out]
        n49 = Release Queue(queue=w110, force destroy? (F)=TRUE, error in (no error)=w109) -> ()  [unwired: 3 out]
      }
      frame "", "Idle" {
        n50 = Unbundle By Name(w125) -> ("ProcessingState"=w123:T10)
        n51 = Equal?(x=w123, y=ProcessingState--enum."Running") -> (x = y?=w121:bool)
        n52 = call "FG - DAQ Error Cluster.vi"("action (Get)"=TD_GetSet_ActionSelect--enum."Get") -> ("error out"=w119:errorcluster)  [unwired: 10 in]
        n53 = Unbundle By Name(w119) -> ("source"=w116:string)
        n54 = case shown="True" w121 {
          tunnel: [w133 w139] -> w127
          tunnel: w126 -> [_ w138]
          tunnel: w124 -> [w131 w136]
          frame False {
            n55 = call <userlib>:"Wait (ms)__ogtk.vi"("error in (no error)"=w131, "milliseconds to wait"=u32 200) -> ("error out"=w133:errorcluster)  [unwired: 8 in, 1 out]
          }
          frame True {
            n56 = call <userlib>:"Wait (ms)__ogtk.vi"("error in (no error)"=w136, "milliseconds to wait"=u32 5) -> ("error out"=w135:errorcluster)  [unwired: 8 in, 1 out]
            n57 = call-poly <vilib>:"Polymorphic - Add States(s) To Queue.vi"("queue in"=w138, "state in"="Action: ReadData", "error in"=w135) -> ("error out"=w139:errorcluster)  [unwired: 9 in, 3 out]
          }
        }
        n58 = Unbundle By Name(w119) -> ("status"=w115:bool)
        n59 = call-poly <userlib>:"Data Changed__ogtk.vi"("String"=w116) -> ("Changed"=w118:bool)
        n60 = Compound Arithmetic op=AND(w115, w118) -> (w117:bool)
        n61 = call <userlib>:"Boolean Trigger__ogtk.vi"("Boolean Input"=w115) -> ("Falling Edge"=w114:bool)  [unwired: 1 in, 1 out]
        n62 = local write "DAQError"(w115) -> ()
        n63 = case shown="True" w117 {
          tunnel: w116 -> [_ w130]
          tunnel: w114 -> [w128 _]
          frame False {
            n64 = case shown="True" w128 {
              frame False {
              }
              frame True {
                n65 = property on="DAQError" class="Bool (strict)"("TipStrip"="") -> ()  [unwired: 2 in, 2 out]
              }
            }
          }
          frame True {
            n66 = property on="DAQError" class="Bool (strict)"("TipStrip"=w130) -> ()  [unwired: 2 in, 2 out]
          }
        }
      }
      frame "------ Macro ------" {
      }
      frame "Macro: Initialize" {
        n67 = call-poly <vilib>:"Polymorphic - Add States(s) To Queue.vi"("queue in"=w145, "states in"="Initialize\n/* some state\n/* another state\nIdle", "error in"=w144) -> ("error out"=w143:errorcluster)  [unwired: 10 in, 2 out]
      }
      frame "Macro: Exit" {
        n68 = call-poly <vilib>:"Polymorphic - Add States(s) To Queue.vi"("queue in"=w150, "states in"="/* some state\n/* another state\nCleanUp\nExit", "error in"=w149) -> ("error out"=w148:errorcluster)  [unwired: 10 in, 2 out]
      }
      frame "------ Action ------" {
      }
      frame "Action: ReadData" {
        n69 = Unbundle By Name(w179) -> ("InvWfmsQ-DT"=w168:T16, "DPAuxDataQ"=w160:T17)
        n70 = call "Create Power Data Plots.vi"("error in (no error)"=w172) -> ("error out"=w163:errorcluster, "DUT3 PowerData"=→"phase3 power data":T19, "DUT2 PowerData"=→"phase2 power data":T19, "DUT1 PowerData"=→"phase1 power data":T19, "DUT4 PowerData"=→"phase4 power data":T19)  [unwired: 6 in]
        n71 = Get Queue Status(queue=w160, error in (no error)=w163) -> (queue out=w169:T17, error out=w162:errorcluster, # elements in queue=→"DP AuxData Size":i32)  [unwired: 1 in, 5 out]
        n72 = Dequeue Element(queue=w169, timeout in ms (-1)=8000, error in (no error)=w162) -> (element=w171:T20[], timed out?=w164:bool, error out=w158:errorcluster)  [unwired: 1 out]
        n73 = Get Queue Status(queue=w168, error in (no error)=w158) -> (queue out=w167:T16, error out=w159:errorcluster, # elements in queue=→"InvWfmsQ DT size":i32)  [unwired: 1 in, 5 out]
        n74 = case shown="False" w164 {
          tunnel: w171 -> [w187 _]
          frame False {
            n75 = for {
              tunnel: w187 -> [w194] mode=indexing
              tunnel: [w193] -> w186
              tunnel: [w192] -> w185
              tunnel: [w191] -> w184 mode=indexing
              tunnel: [w190] -> w183
              tunnel: [w189] -> w181
              tunnel: [w188] -> w180
              n76 = Unbundle(w194) -> ("Raw ESR sum"=w193:dbl, "Inv 1 ON?"=w190:bool, "Average scaled ESR sum"=w189:dbl, "Inv 1 over threshold?"=w192:bool, "Inv 1 ESR"=w191:T21, "Max ESR"=w188:dbl)  [unwired: 1 out]
            }
            "Raw  ESR" <- w186
            "Inverter ESR status" <- w185
            "Scaled & avgd ESR" <- w181
            "Max ESR" <- w180
            n77 = case shown="True" w183 {
              tunnel: w184 -> [_ w197]
              tunnel: ["OFF - NO DATA" ("Inverter 1 state:") "RUNNING"] -> w182
              frame False {
              }
              frame True {
                "Equivalent Series Resistance (ESR)" <- w197
              }
            }
            "Inverter State" <- w182
          }
          frame True {
          }
        }
        n78 = Dequeue Element(queue=w167, timeout in ms (-1)=8000, error in (no error)=w159) -> (element=w178:T22, timed out?=w165:bool, error out=w177:errorcluster)  [unwired: 1 out]
        n79 = case shown="False" w165 {
          tunnel: w178 -> [w207 _]
          tunnel: w177 -> [w206 w208]
          tunnel: [w199 w208] -> w173
          frame False {
            n80 = call "Create Graph Plot Arrays.vi"("error in"=w206, "InverterWaveforms"=w207) -> ("error out"=w199:errorcluster, "DUT1 60 Hz V and I"=→"DUT1 I-V":waveform(dbl)[], "Iouts 60Hz"=→"Iout 60Hz":waveform(dbl)[], "DUT4 60 Hz V and I"=→"DUT4 I-V":waveform(dbl)[], "DUT2 60 Hz V and I"=→"DUT2 I-V":waveform(dbl)[], "Iout ripples"=→"Iout ripple":waveform(dbl)[], "DUT3 60 Hz V and I"=→"DUT3 I-V":waveform(dbl)[], "Iin ripples"=→"Iin ripple":waveform(dbl)[])  [unwired: 2 in]
          }
          frame True {
          }
        }
        n81 = call-poly <userlib>:"Filter Error Codes__ogtk.vi"("Error In"=w173, "Error Codes to Filter"=i32[] [1122]) -> ("Error Out"=w156:errorcluster)  [unwired: 7 in, 2 out]
      }
      frame "Action: Wait" {
        n82 = Scan From String(format string="%d", input string=w211, error in=w210, default 1=u32 0) -> (error out=w209:errorcluster, output 1=w215:u32)  [unwired: 1 in, 2 out]
        n83 = call <userlib>:"Wait (ms)__ogtk.vi"("error in (no error)"=w209, "milliseconds to wait"=w215) -> ("error out"=w213:errorcluster)  [unwired: 8 in, 1 out]
      }
      frame "Action: UpdateSMData" {
        n84 = Match Pattern(string=w224, regular expression=":") -> (before substring=w226:string, after substring=w217:string)  [unwired: 1 in, 2 out]
        n85 = case shown="\"ProcessingState\"" w226 {
          tunnel: w223 -> [_ w235]
          tunnel: w222 -> [_ _]
          tunnel: w221 -> [w227 w234]
          tunnel: [w227 w233] -> w220
          tunnel: w219 -> [w228 w232]
          tunnel: [w228 w231] -> w218
          tunnel: w217 -> [_ _]
          frame Default {
            # "#NOTE:\noptionally add error here."
          }
          frame "ProcessingState" {
            n86 = Variant To Data(error in=w232, type=ProcessingState--enum."Idle" ("y"), Variant=w235) -> (data=w229:T10, error out=w231:errorcluster)
            n87 = Bundle By Name(cluster=w234, "ProcessingState"=w229) -> (w233:T12)
          }
        }
      }
    }
  }
  n88 = while {
    shift-right: [w246] -> _
    shift-left: w4 -> [w245]
    shift-right: [w249] -> w3
    shift-left: w6 -> [w244]
    shift-right: [w248] -> _
    shift-left: w9 -> [w250]
    shift-right: [w243] -> _
    shift-left: _ -> [w242]
    tunnel: w8 -> [w240]
    tunnel: w7 -> [w239]
    tunnel: w1 -> [w238]
    stop <- w247 stop-if-true
    n89 = call <vilib>:"Parse State Queue__JKI_lib_State_Machine.vi"("State Queue"=w250, "Error In (no error)"=w244) -> ("Remaining States"=w252:string, "Current State"=w237:string, "Arguments"=w251:string)  [unwired: 11 in]
    n90 = feedback #1(w238) -> (w236:string)
    n91 = feedback-in #1(w237) -> ()
    n92 = case shown="\"Action: View Inverter Param Values\"" w237 {
      selector: w237 -> [w254 _ _ _ _ _ _ _ _ _ _ _ _ _ _ _ _ _ _ _ _ _ _ _ _ _ _ _ _ _ _ _ _]
      tunnel: w252 -> [w258 w273 w279 w312 w704 w717 w725 w738 w742 w747 w760 w789 w796 w801 w817 w832 w846 w855 w883 w895 w902 w918 w970 w976 w995 w1000 w1016 w1044 w1076 w1099 w1116 w1128 w1137]
      tunnel: w251 -> [_ _ _ _ _ _ _ _ _ _ _ _ _ _ _ _ _ _ _ _ w897 w913 _ _ _ _ _ _ _ _ _ w1118 _]
      tunnel: w245 -> [w256 w270 w274 w310 w701 w708 w722 w735 w741 w744 w749 w780 w791 w798 w810 w823 w843 w849 w873 w885 w900 w911 w967 w973 w992 w997 w1012 w1030 w1073 w1096 w1113 w1126 w1134]
      tunnel: [w260 errorcluster {"status"=FALSE, "code"=0, "source"=""} ("error out") w277 w309 w702 w714 w718 w736 w739 w745 w750 w787 w792 w799 w811 w818 w840 w848 w881 w891 w898 w915 w968 w974 w993 w998 w1014 w1019 w1054 w1086 w1108 w1119 w1129] -> w249
      tunnel: w244 -> [w259 w266 w277 w308 w702 w714 w719 w726 w739 w745 w756 w787 w793 w799 w808 w825 w839 w847 w881 w892 w899 w916 w968 w974 w993 w998 w1014 w1042 w1053 w1085 w1106 w1120 w1130]
      tunnel: [w257 w272 w278 w311 w703 w716 w724 w738 w742 w746 w759 w788 w795 w800 w816 w831 w845 w854 w882 w894 w901 w917 w969 w975 w994 w999 w1015 w1043 w1075 w1098 w1115 w1127 w1136] -> w248
      tunnel: [_ _ TRUE _ _ _ _ _ _ _ _ _ _ _ _ _ _ _ _ _ _ _ _ _ _ _ _ _ _ _ _ _ _] -> w247
      tunnel: [w256 w270 w274 w307 w701 w715 w722 w735 w741 w744 w749 w785 w791 w798 w810 w824 w843 w849 w873 w886 w900 w911 w967 w973 w992 w997 w1012 w1030 w1073 w1096 w1113 w1126 w1134] -> w246
      tunnel: [w253 w268 w275 w305 w700 w705 w723 w737 w740 w743 w758 w784 w790 w797 w815 w830 w844 w853 w874 w893 w896 w912 w966 w972 w988 w996 w1013 w1041 w1074 w1097 w1114 w1125 w1135] -> w243
      tunnel: w242 -> [w253 w268 w275 w305 w700 w705 w723 _ w740 w743 w758 w784 w790 w797 w815 w830 w844 w853 w874 w893 w896 w912 w966 w972 w988 w996 w1013 w1041 w1074 w1097 w1114 w1125 w1135]
      tunnel: 200 ("Timeout") -> [_ _ _ w306 _ _ _ _ _ _ _ _ _ _ _ _ _ _ _ _ _ _ _ _ _ _ _ _ _ _ _ _ _]
      tunnel: w240 -> [_ _ _ _ _ _ _ _ _ _ _ _ _ _ _ _ _ _ _ _ _ _ _ w971 _ _ _ _ _ _ _ _ _]
      tunnel: w239 -> [_ _ _ _ _ _ _ _ _ _ _ _ _ _ _ _ _ _ _ _ _ _ _ _ w981 _ _ _ _ _ _ _ _]
      tunnel: w236 -> [_ w265 _ _ _ _ _ _ _ _ _ _ _ _ _ _ _ _ _ _ _ _ _ _ _ _ _ _ _ _ _ _ _]
      frame Default {
        w263 = 42 items=["No error", "Argument error", "Memory is full", "Out of zone", "End of file", "File already open", "Generic file I/O error", "File not found", "File permission error", "Disk is full", "Duplicate path", "Too many files open", "System feature not enabled", "Resource file not found", "Cannot add resource", "Resource not found", "Image not found", "Image memory error", "Pen does not exist", "Config type invalid", "Config token not found", "Config parse error", "Config memory error", "Bad external code format", "Bad external code offset", "External code not present", "Null window", "Destroy window error", "Null menu", "Print aborted", "Bad print record", "Print driver error", "Windows error during printing", "Memory error during printing", "Print dialog error", "Generic print error", "Invalid device refnum", "Device not found", "Device parameter error", "Device unit error", "Cannot open device", "Device call aborted", "Generic error", "Cancelled by user", "Object ID too low", "Object ID too high", "Object not in heap", "Unknown heap", "Unknown object (invalid DefProc)", "Unknown object (DefProc not in table)", "Message out of range", "Invalid (null) method", "Unknown message", "Manager call not supported", "Bad address", "Network operation in progress", "Network operation timed out", "Connection is busy", "Network attribute not supported", "Network error", "Address in use", "System out of memory", "Connection aborted", "Connection refused", "Not connected", "Already connected", "Connection closed", "Initialization error (interapplication manager)", "Bad occurrence", "Wait on unbound occurrence handler", "Occurrence queue overflow", "Datalog type conflict", "Unused", "Unrecognized type (interapplication manager)", "Memory corrupt", "Failed to make temporary DLL", "Old CIN version", "Drag socket not found", "Failed to load drop-object", "Failed to register OLE object", "Failed to release OLE object", "Format specifier type mismatch", "Unknown format specifier", "Too few format specifiers", "Too many format specifiers", "Scan failed", "Newer CIN version", "Error converting to variant", "Runtime menu error", "Password tampered", "Variant attribute not found", "Incompatible variant data type", "Event data is not available", "Event Store is not present", "Occurrence is not found", "Event Queue is not created", "Event info is not available", "Refnum passed is NULL", "Error retrieving Class GUID", "Error retrieving CoClass GUID", "Error retrieving TypeLib GUID.", "Bad built application magic bytes.", "Specific driver is different from the specific driver associated with the Logical Name.", "There is no session opened to the class driver.", "Max Error", "MAX - Error with config objects", "MAX - Error loading configuration", "MAX - Group not supported"]
        # "Current State"
        n93 = Format Into String(format string="Software Exception: Unhandled State \"%s\"." ("message"), error in=w259, w254) -> (resulting string=w262:string, error out=w261:errorcluster)  [unwired: 1 in]
        n94 = call <vilib>:"Error Cluster From Error Code.vi"("show call chain? (False)"=TRUE, "error in (no error)"=w261, "error message (\"\")"=w262, "error code (0)"=w263) -> ("error out"=w260:errorcluster)  [unwired: 5 in]
        n95 = call <vilib>:"Add State(s) to Queue__JKI_lib_State_Machine.vi"("State(s) in (\"\")"=w258) -> ("States Out"=w257:string)  [unwired: 14 in]
      }
      frame "Error Handler" {
        n96 = call "General Error Handler - show previous state.vi"("error in (no error)"=w266, "Previous State"=w265, "Loop Select"=enum16{"Event Loop -", "Async Loop -"}."Event Loop -") -> ()  [unwired: 7 in, 2 out]
        n97 = call <vilib>:"Add State(s) to Queue__JKI_lib_State_Machine.vi"("State(s) in Front (\"\")"="/* Post Error States", "State(s) in (\"\")"=w273) -> ("States Out"=w272:string)  [unwired: 13 in]
      }
      frame "Exit" {
        n98 = disable-structure shown="Enabled" {
          disable-tunnel: w274 -> [_ w299]
          frame Disabled {
            n99 = Unbundle By Name() -> (w280:T41, "RuntimeSystem?"=w283, "Core.Current VI Reference"=w281, "Rect"=w282)
            n100 = case shown="False" w283 {
              tunnel: w281 -> [w297 w298]
              tunnel: w282 -> [w296 _]
              tunnel: [w295 w298] -> w289
              frame False {
                n101 = property class="VI"(reference=w297, "Front Panel.PanelBounds"=w296, "Front Panel.ShowMenuBar"=TRUE) -> (reference out=w295:refnum<vi>, error out=w291:errorcluster)  [unwired: 1 in]
                n102 = Current VI's Path() -> (path=w294:path)
                n103 = call <vilib>:"show scrollbars v2.vi"("mode (read)"=enum16{"read", "write", "toggle"}."write", "error in (no error)"=w291, "ShowScrollbars?"=TRUE, "vi path"=w294) -> ()  [unwired: 3 in, 2 out]
              }
              frame True {
              }
            }
            n104 = Close Reference(reference=w289) -> (error out=w287:errorcluster)  [unwired: 1 in]
            n105 = call <userlib>:"Clear All Errors__ogtk.vi"("Error In"=w287) -> ("Error Out"=w288:errorcluster)  [unwired: 3 in]
            n106 = call <vilib>:"Delete ALL Dynamic CVT Data.vi"("error in (no error)"=w288) -> ("error out"=w284:errorcluster, "dCVT DVR out"=w285:T18, "dCVT DVR"=w286:T18)  [unwired: 8 in]
            n107 = call <vilib>:"Destroy Dynamic CVT Reference.vi"("error in (no error)"=w284, "dCVT DVR"=w285) -> ()  [unwired: 8 in, 2 out]
          }
          frame Enabled {
            n108 = Unbundle By Name(w299) -> ("Core.Current VI Reference"=w300:refnum<vi>)  [unwired: 1 out]
            n109 = Close Reference(reference=w300) -> (error out=w301:errorcluster)  [unwired: 1 in]
            n110 = call <userlib>:"Clear All Errors__ogtk.vi"("Error In"=w301) -> ()  [unwired: 3 in, 1 out]
            n111 = Current VI's Path() -> (path=w304:path)
            n112 = call <vilib>:"show scrollbars v2.vi"("mode (read)"=enum16{"read", "write", "toggle"}."write", "ShowScrollbars?"=TRUE, "vi path"=w304) -> ()  [unwired: 4 in, 2 out]
          }
        }
        n113 = call <vilib>:"Add State(s) to Queue__JKI_lib_State_Machine.vi"("State(s) in (\"\")"=w279) -> ("States Out"=w278:string)  [unwired: 14 in]
      }
      frame "", "Event Structure", "Idle" {
        n114 = event shown="[19] \"SelectInverter\", \"Trigger SelectInverter Event\": Value Change" {
          selector: w305 -> [_ _ _ _ _ _ _ _ _ _ _ _ _ _ _ _ _ _ _ _ _ _ _ _ _ _ _ _ _ _ _ _]
          dyn-events: _ -> [_ _ _ _ _ _ _ _ _ _ _ _ _ _ _ _ _ _ _ _ _ _ _ _ _ _ _ _ _ _ _ _]
          timeout: w306 -> [_ _ _ _ _ _ _ _ _ _ _ _ _ _ _ _ _ _ _ _ _ _ _ _ _ _ _ _ _ _ _ _]
          tunnel: w312 -> [w316 w325 w332 w335 w347 w354 w365 w371 w377 w384 w391 w404 w419 w438 w450 w456 w484 w498 w503 w523 w537 w544 w564 w580 w595 w601 w604 w620 w669 w677 w685 w699]
          tunnel: [w315 w324 w331 w334 w347 w354 w365 w371 w377 w384 w391 w404 w419 w438 w450 w456 w484 w498 w503 w523 w537 w545 w564 w580 w595 w601 w603 w619 w669 w677 w685 w699] -> w311
          tunnel: w310 -> [w313 w321 w329 w337 w345 w351 w363 w370 w376 w383 w390 w403 w416 w437 w449 w454 w482 w496 w501 w522 w535 w541 w557 w579 w594 w600 w607 w609 w663 w672 w680 w696]
          tunnel: [w314 w323 w330 w338 w344 w350 w360 w368 w374 w379 w387 w400 w413 w436 w447 w455 w483 w497 w502 w511 w536 w546 w563 w577 w592 w598 w608 w617 w668 w676 w684 w694] -> w309
          tunnel: w308 -> [w314 w323 w330 w338 w344 w349 w359 w367 w375 w378 w388 w401 w412 w431 w446 w455 w483 w497 w502 w512 w536 w547 w563 w576 w591 w597 w608 w616 w668 w676 w684 w693]
          tunnel: [w313 w321 w329 w337 w345 w351 w363 w370 w376 w383 w390 w403 w416 w437 w449 w454 w482 w496 w501 w522 w535 w542 w558 w579 w594 w600 w606 w611 w664 w673 w681 w697] -> w307
          event Timeout {
            n115 = event-data() -> ()  [unwired: 1 in, 1 out]
            n116 = call <vilib>:"Add State(s) to Queue__JKI_lib_State_Machine.vi"("State(s) in (\"\")"=w316) -> ("States Out"=w315:string)  [unwired: 14 in]
          }
          event "Exit": Value Change {
            n117 = event-data() -> ()  [unwired: 1 in, 6 out]
            n118 = call <vilib>:"Three Button Dialog.vi"("Window Title (\"\")"="SYSTEM: Terminate" ("Window Title (\"\")"), "Center Button Text (\"No\")"="", "message"="Terminate Program?") -> ("Which Button?"=w317:T34)  [unwired: 8 in]
            n119 = case shown="Default" w317 {
              tunnel: [_ "Macro: Exit"] -> w322
              frame Default {
              }
              frame "Left Button" {
              }
            }
            n120 = call <vilib>:"Add State(s) to Queue__JKI_lib_State_Machine.vi"("State(s) in Front (\"\")"=w322, "State(s) in (\"\")"=w325) -> ("States Out"=w324:string)  [unwired: 13 in]
          }
          event Panel Close? {
            n121 = event-data() -> ()  [unwired: 1 in, 1 out]
            n122 = event-data("Discard?"=TRUE) -> ()  [unwired: 1 in, 1 out]
            n123 = call <vilib>:"Add State(s) to Queue__JKI_lib_State_Machine.vi"("State(s) in Front (\"\")"="Macro: Exit", "State(s) in (\"\")"=w332) -> ("States Out"=w331:string)  [unwired: 13 in]
          }
          event Menu Selection (User) {
            n124 = event-data() -> ("ItemTag"=w336:string)  [unwired: 1 in, 2 out]
            n125 = case shown="\"Launch ESR Gain & Offset Explorer\"" w336 {
              tunnel: ["" "Macro: Exit" "UI: Launch TDMS Viewer" "UI: Show About Dialog" "UI: Launch ESR Gain&Offset Explorer"] -> w333
              frame Default {
              }
              frame "Exit" {
              }
              frame "TDMS File Viewer" {
              }
              frame "About" {
              }
              frame "Launch ESR Gain & Offset Explorer" {
              }
            }
            n126 = call <vilib>:"Add State(s) to Queue__JKI_lib_State_Machine.vi"("State(s) in Front (\"\")"=w333, "State(s) in (\"\")"=w335) -> ("States Out"=w334:string)  [unwired: 13 in]
          }
          event "SystemError": Mouse Down {
            # "Reset system error indicator when mouse down on the indicator"
            n127 = event-data() -> ()  [unwired: 1 in, 8 out]
            n128 = local write "SystemError"(FALSE ("SystemError")) -> ()
          }
          event "DAQError": Mouse Down {
            # "Reset system error indicator when mouse down on the indicator"
            n129 = event-data() -> ()  [unwired: 1 in, 8 out]
            n130 = Unbundle By Name(w351) -> ("Dependency.DAQ"=w352:refnum<class "DAQ_Engine.lvclass">)
            n131 = call "Generate Async Cmd Event.vi"("error in (no error)"=w349, "AsyncCmd"=AsynCmd_DAQ_Engine--enum."DAQ.ClearDAQError", "DAQ_Engine in"=w352) -> ("error out"=w350:errorcluster)  [unwired: 7 in, 1 out]
            n132 = local write "DAQError"(FALSE ("SystemError")) -> ()
          }
          event "UpdateDAQSettings": Value Change {
            n133 = event-data() -> ()  [unwired: 1 in, 1 out]
            n134 = Unbundle By Name(w363) -> ("Dependency.DAQ"=w362:refnum<class "DAQ_Engine.lvclass">)
            n135 = Bundle By Name(cluster=T5 {"Data Rate 9775"=3.0, "Data Rate 9215"=1200000.0, "Samples RMS 9215"=480000, "Samples RMS 9775"=3} ("MeasSet"), "Data Rate 9775"="Data Rate 9775(S/s)", "Data Rate 9215"="Data Rate 9215 (S/s)", "Samples RMS 9215"="Samples RMS 9215", "Samples RMS 9775"="Samples RMS 9775") -> (w361:T5)
            "MeasSet" <- w361
            n136 = call "CMD SetMeasConfig.vi"("error in (no error)"=w359, "MeasSet"=w361, "DAQ_Engine in"=w362) -> ("error out"=w360:errorcluster)  [unwired: 7 in, 1 out]
          }
          event Value Change {
            n137 = event-data() -> ("NewVal"=w366:T3)  [unwired: 1 in]
            n138 = Unbundle By Name(w370) -> ("Dependency.DAQ"=w369:refnum<class "DAQ_Engine.lvclass">)
            n139 = call "CMD SetAcqMode.vi"("error in (no error)"=w367, "Acqusition Mode"=w366, "DAQ_Engine in"=w369) -> ("error out"=w368:errorcluster)  [unwired: 7 in, 1 out]
          }
          event "cRIO Error\nReporting Mode": Value Change {
            n140 = event-data() -> ("NewVal"=w372:i32)  [unwired: 1 in]
            n141 = Unbundle By Name(w376) -> ("Dependency.DAQ"=w373:refnum<class "DAQ_Engine.lvclass">)
            n142 = call "CMD DAQ Error Reporting Mode.vi"("error in (no error)"=w375, "DAQ Error\nReporting Mode"=w372, "DAQ_Engine in"=w373) -> ("error out"=w374:errorcluster)  [unwired: 7 in, 1 out]
          }
          event "DAQEnDis": Value Change {
            # "toggle present state"
            n143 = event-data() -> ()  [unwired: 1 in, 1 out]
            n144 = Unbundle By Name(w383) -> ("DAQEnabled"=w381:bool, "Dependency.DAQ"=w382:refnum<class "DAQ_Engine.lvclass">)
            n145 = Not(x=w381) -> (.not. x?=w380:bool)
            n146 = call "CMD StartStopDAQ.vi"("error in (no error)"=w378, "DAQEnable"=w380, "DAQ_Engine in"=w382) -> ("error out"=w379:errorcluster)  [unwired: 7 in, 1 out]
          }
          event "LogEnDis": Value Change {
            # "toggle present state"
            n147 = event-data() -> ()  [unwired: 1 in, 1 out]
            n148 = Unbundle By Name(w390) -> ("LoggingEnabled"=w389:bool, "Dependency.Log_Engine"=w386:refnum<class "Log_Engine.lvclass">)
            n149 = Not(x=w389) -> (.not. x?=w385:bool)
            n150 = case shown="False" w385 {
              tunnel: w388 -> [w393 w397]
              tunnel: [w392 w396] -> w387
              tunnel: w386 -> [w394 w395]
              frame False {
                n151 = call "CMD StopESRLog.vi"("error in (no error)"=w393, "Log_Engine in"=w394) -> ("error out"=w392:errorcluster)  [unwired: 8 in, 1 out]
              }
              frame True {
                n152 = call "CMD StartESRLog.vi"("error in (no error)"=w397, "Log_Engine in"=w395) -> ("error out"=w396:errorcluster)  [unwired: 8 in, 1 out]
              }
            }
          }
          event "TDMSEnDis": Value Change {
            # "toggle present state"
            n153 = event-data() -> ()  [unwired: 1 in, 1 out]
            n154 = Unbundle By Name(w403) -> ("TDMS Enabled"=w402:bool, "Dependency.Log_Engine"=w399:refnum<class "Log_Engine.lvclass">)
            n155 = Not(x=w402) -> (.not. x?=w398:bool)
            n156 = case shown="False" w398 {
              tunnel: w401 -> [w406 w410]
              tunnel: [w405 w409] -> w400
              tunnel: w399 -> [w407 w408]
              frame False {
                n157 = call "CMD StopLog.vi"("error in (no error)"=w406, "Log_Engine in"=w407) -> ("error out"=w405:errorcluster)  [unwired: 8 in, 1 out]
              }
              frame True {
                n158 = call "CMD StartLog.vi"("error in (no error)"=w410, "Log_Engine in"=w408) -> ("error out"=w409:errorcluster)  [unwired: 8 in, 1 out]
              }
            }
          }
          event "ESR scaling", "Dummy Vrms", "UseDummyVrms", "Settings.Signal scaling": Value Change {
            # "These are used in Process for data processing"
            n159 = event-data() -> ("CtlRef"=w418:refnum<vi>, "NewVal"=w411:variant)  [unwired: 1 in]
            n160 = Unbundle By Name(w416) -> ("Self Reference"=w415:refnum<class "Main.lvclass">)
            n161 = property class="Ctl"(reference=w418, error in=w412) -> (error out=w414:errorcluster, "Label.Text"=w417:string)  [unwired: 1 out]
            n162 = call "Fire UpdateControlValue Event.vi"("error in (no error)"=w414, "vData"=w411, "Control Label"=w417, "Main in"=w415) -> ("error out"=w413:errorcluster)  [unwired: 6 in, 1 out]
          }
          event "StartProcessing": Value Change {
            w428 = T27 {"MinCurrThreshold"=1.5, "NumPF RdsToAvg"=10, "ESR alarm threshhold (%)"=200.0, "# readings to average"=40}  # ProcessInitParams
            w434 = T26 {"Inverter ID"=""}  # InverterInfo
            n163 = event-data() -> ()  [unwired: 1 in, 1 out]
            n164 = Unbundle By Name(w437) -> ("Self Reference"=w435:refnum<class "Main.lvclass">, "ProcessingState"=w433:T10)
            n165 = Not Equal?(x=w433, y=ProcessingState--enum."Running") -> (x != y?=w430:bool)
            n166 = Bundle By Name(cluster=w428, "MinCurrThreshold"="MinCurrThreshold", "NumPF RdsToAvg"="NumPF RdsToAvg", "ESR alarm threshhold (%)"="ESR alarm threshhold (%)", "# readings to average"="# readings to average") -> (w425:T27)
            n167 = Bundle By Name(cluster=w434, "Inverter ID"="Inverter ID") -> (w427:T26)
            n168 = Bundle(cluster=T25 {"InverterInfo"={"Inverter ID"=""}, "ProcessInitParams"={"MinCurrThreshold"=1.5, "NumPF RdsToAvg"=10, "ESR alarm threshhold (%)"=200.0, "# readings to average"=40}} ("StartProcInitParams"), "InverterInfo"=w427, "ProcessInitParams"=w425) -> (w426:T25)
            n169 = case shown="True" w430 {
              tunnel: w431 -> [w440 w445]
              tunnel: [w441 w444] -> w436
              tunnel: w435 -> [_ w443]
              tunnel: w426 -> [_ w442]
              frame False {
                n170 = call "Dialog Box Timeout v2.vi"("Error In"=w440, "Message"="Data Processing Already Running") -> ("Error Out"=w441:errorcluster)  [unwired: 9 in]
              }
              frame True {
                n171 = call "CMD StartProcessing.vi"("error in (no error)"=w445, "StartProcInitParams"=w442, "Main in"=w443) -> ("error out"=w444:errorcluster)  [unwired: 7 in, 1 out]
              }
            }
          }
          event "StopProcessing": Value Change {
            n172 = event-data() -> ()  [unwired: 1 in, 1 out]
            n173 = Unbundle By Name(w449) -> ("Self Reference"=w448:refnum<class "Main.lvclass">)
            n174 = call "CMD StopProcessing.vi"("error in (no error)"=w446, "Main in"=w448) -> ("error out"=w447:errorcluster)  [unwired: 8 in, 1 out]
          }
          event "DataPg_button", "Page2Pg_button", "ConfigPg_button", "SettingsPg_button": Value Change {
            n175 = event-data() -> ("NewVal"=w451:bool, "CtlRef"=w453:refnum<vi>)  [unwired: 1 in]
            n176 = property class="Bool (strict)"(reference=w453) -> ("Label.Text"=w452:string)  [unwired: 1 in, 2 out]
            n177 = case shown="True" w451 {
              selector: w451 -> [_ w461]
              tunnel: w452 -> [_ w463]
              frame False {
              }
              frame True {
                n178 = case shown="\"SettingsPg_button\"" w463 {
                  tunnel: w461 -> [w466 w468 w472 w474]
                  tunnel: [w466 w469 w471 w475] -> w462
                  tunnel: [w465 w468 w471 w475] -> w460
                  tunnel: [w465 w469 w472 w474] -> w459
                  tunnel: [w465 w469 w471 w474] -> w458
                  tunnel: [T1."Data" ("LeftPanelTab") T1."InverterSel" ("LeftPanelTab") T1."Config" ("LeftPanelTab") T1."Settings" ("LeftPanelTab")] -> w457
                  frame "DataPg_button", Default {
                    w465 = FALSE
                  }
                  frame "Page2Pg_button" {
                    w469 = FALSE
                  }
                  frame "ConfigPg_button" {
                    w471 = FALSE
                  }
                  frame "SettingsPg_button" {
                    w475 = FALSE
                  }
                }
                n179 = local write "DataPg_button"(w462) -> ()
                n180 = local write "Page2Pg_button"(w460) -> ()
                n181 = local write "ConfigPg_button"(w459) -> ()
                n182 = local write "SettingsPg_button"(w458) -> ()
                n183 = local write "LeftPanelTab"(w457) -> ()
              }
            }
          }
          event "Show_ESR_Data", "Show_TimeSeries_Data", "Show_PowerFactor_Data": Value Change {
            n184 = event-data() -> ("CtlRef"=w481:refnum<vi>)  [unwired: 1 in]
            n185 = property class="Bool"(reference=w481) -> ("Label.Text"=w480:string)  [unwired: 1 in, 2 out]
            n186 = case shown="\"Show_PowerFactor_Data\"" w480 {
              tunnel: [TRUE w490 w493] -> w479
              tunnel: [w487 TRUE w493] -> w478
              tunnel: [w487 w490 TRUE] -> w477
              tunnel: [T6."ESRData" ("MainPanelTab") T6."TimeSeriesData" ("MainPanelTab") T6."PowerFactorData" ("MainPanelTab")] -> w476
              frame "Show_ESR_Data", Default {
                w487 = FALSE
              }
              frame "Show_TimeSeries_Data" {
                w490 = FALSE
              }
              frame "Show_PowerFactor_Data" {
                w493 = FALSE
              }
            }
            n187 = local write "Sel_ESR_Data"(w479) -> ()
            n188 = local write "Sel_TimeSeries_Data"(w478) -> ()
            n189 = local write "Sel_PowerFactor_Data"(w477) -> ()
            n190 = local write "MainPanelTab"(w476) -> ()
          }
          event "toggle MainTabDbgPg": Value Change {
            w495 = FALSE
            n191 = event-data() -> ()  [unwired: 1 in, 3 out]
            n192 = local write "MainPanelTab"(T6."DebugPage" ("MainPanelTab")) -> ()
            n193 = local write "Sel_ESR_Data"(w495) -> ()
            n194 = local write "Sel_TimeSeries_Data"(w495) -> ()
            n195 = local write "Sel_PowerFactor_Data"(w495) -> ()
          }
          event "toggle scrollbars": Value Change {
            n196 = event-data() -> ()  [unwired: 1 in, 3 out]
            n197 = Current VI's Path() -> (path=w500:path)
            n198 = call <vilib>:"show scrollbars v2.vi"("mode (read)"=enum16{"read", "write", "toggle"}."toggle", "vi path"=w500) -> ()  [unwired: 5 in, 2 out]
          }
          event "SelectInverter", "Trigger SelectInverter Event": Value Change {
            n199 = event-data() -> ()  [unwired: 1 in, 1 out]
            n200 = Unbundle By Name(w522) -> ("Self Reference"=w521:refnum<class "Main.lvclass">)
            n201 = property class="Main.lvclass"(reference=w521, error in=w512) -> (reference out=w515:refnum<class "Main.lvclass">, error out=w513:errorcluster, "Accessors:InvLUTDict*"=w520:T18, "Accessors:CurrInverter*"=w516:T37[])
            n202 = for {
              tunnel: w520 -> [w529]
              tunnel: "Selected Inverter" -> [w528] mode=indexing
              tunnel: [w527] -> w518
              tunnel: w516 -> [w525] mode=indexing
              shift-right: [w526] -> w517
              shift-left: w513 -> [w524]
              n203 = call <vilib>:"Get Dynamic CVT Data.vi"("error in (no error)"=w524, "value"=w525, "DataName"=w528, "dCVT DVR"=w529) -> ("error out"=w526:errorcluster, "value"=w527:variant)  [unwired: 4 in, 2 out]
            }
            n204 = Variant To Data(error in=w517, type=w516, Variant=w518) -> (data=w504:T37[], error out=w514:errorcluster)
            n205 = property class="Main.lvclass"(reference=w515, error in=w514, "Accessors:CurrInverter*"=w504) -> (reference out=w509:refnum<class "Main.lvclass">, error out=w507:errorcluster)
            n206 = call "Fire Private Event.vi"("error in (no error)"=w507, "vData"=w504, "PrivAsync"=PrivateAsynEv_Main--enum."PrivMain.CurrInverterUpdated", "Main in"=w509) -> ("error out"=w506:errorcluster, "Main out"=w508:refnum<class "Main.lvclass">)  [unwired: 6 in]
            n207 = call "Generate Async Msg Event.vi"("error in (no error)"=w506, "vData"=w504, "AsyncMsg"=AsynMsg_Main--enum."Main.CurrInverterUpdated", "Main in"=w508) -> ("error out"=w511:errorcluster)  [unwired: 6 in, 1 out]
            n208 = case shown="No Error" w511 {
              frame No Error {
                n209 = local write "InvSelLED"(TRUE ("InvSelLED")) -> ()
              }
              frame Error {
              }
            }
          }
          event "Inverter List": Value Change {
            n210 = event-data() -> ()  [unwired: 1 in, 6 out]
            n211 = local read "Inverter List"() -> (w534:i32[])
            n212 = property on="Inverter List" class="LstBox (strict)"() -> ("Item Names"=w533:string[])  [unwired: 2 in, 2 out]
            n213 = for {
              tunnel: w534 -> [w540] mode=indexing
              tunnel: w533 -> [w539]
              tunnel: [w538] -> w532 mode=indexing
              n214 = Index Array(array=w539, index=w540) -> (element=w538:string)
            }
            n215 = local write "InvSelLED"(FALSE ("InvSelLED")) -> ()
            n216 = local write "Selected Inverter"(w532) -> ()
          }
          event "Inverter List": Shortcut Menu Selection (User) {
            n217 = event-data() -> ("ItemTag"=w548:string)  [unwired: 1 in, 7 out]
            n218 = case shown="\"View Selected Inverter Param Values\"" w548 {
              tunnel: w547 -> [w550 w553 w556]
              tunnel: [w550 w553 w556] -> w546
              tunnel: [_ "Action: View Inverter Param Values" "Action: Open Inverter LUT DB Editor"] -> w543
              tunnel: w541 -> [w549 w551 w555]
              tunnel: [w549 w551 w555] -> w542
              frame Default {
              }
              frame "View Selected Inverter Param Values" {
              }
              frame "Open Inverter LUT DB Editor" {
              }
            }
            n219 = call <vilib>:"Add State(s) to Queue__JKI_lib_State_Machine.vi"("State(s) in Front (\"\")"=w543, "State(s) in (\"\")"=w544) -> ("States Out"=w545:string)  [unwired: 13 in]
          }
          event "TitleBar", "TitleBar Text", "TitleBar AppVerText": Mouse Down? {
            n220 = event-data() -> ("Button"=w561:u16)  [unwired: 1 in]
            n221 = Unbundle By Name(w557) -> ("Core.Current VI Reference"=w560:refnum<vi>, "MenuBarShown?"=w559:bool)
            n222 = case shown="2" w561 {
              tunnel: w560 -> [_ w567 w572]
              tunnel: w559 -> [_ _ w569]
              tunnel: w557 -> [w565 w566 w571]
              tunnel: [w565 w566 w570] -> w558
              frame 0, Default {
              }
              frame 1 {
                n223 = call "Start Window Drag.vi"("VI Ref (calling VI)"=w567) -> ()  [unwired: 9 in, 2 out]
              }
              frame 2 {
                n224 = Not(x=w569) -> (.not. x?=w568:bool)
                n225 = property class="VI"(reference=w572, "Front Panel.ShowMenuBar"=w568) -> ()  [unwired: 1 in, 2 out]
                n226 = Bundle By Name(cluster=w571, "MenuBarShown?"=w568) -> (w570:T12)
              }
            }
            n227 = event-data("Discard?"=TRUE) -> ()  [unwired: 1 in, 1 out]
          }
          event "StoreESR BLine", "UseSavedESR BLine": Value Change {
            n228 = event-data() -> ()  [unwired: 1 in, 1 out]
            n229 = Unbundle By Name(w579) -> ("Self Reference"=w578:refnum<class "Main.lvclass">)
            n230 = Compound Arithmetic op=OR("StoreESR BLine", "UseSavedESR BLine") -> (w575:bool)
            n231 = case shown="True" w575 {
              tunnel: w578 -> [_ w585]
              tunnel: [w581 w584] -> w577
              tunnel: w576 -> [w581 w583]
              frame False {
              }
              frame True {
                n232 = call "Fire Private Event.vi"("error in (no error)"=w583, "PrivAsync"=PrivateAsynEv_Main--enum."PrivMain.UpdateStoreUseESRBaseline", "Main in"=w585) -> ("error out"=w584:errorcluster)  [unwired: 7 in, 1 out]
              }
            }
          }
          event "set alarm", "reset alarm": Value Change {
            n233 = event-data() -> ("CtlRef"=w590:refnum<vi>)  [unwired: 1 in]
            n234 = property class="Bool"(reference=w590) -> ("Label.Text"=w589:string)  [unwired: 1 in, 2 out]
            n235 = Equal?(x=w589, y="set alarm") -> (x = y?=w587:bool)
            n236 = Unbundle By Name(w594) -> ("Self Reference"=w593:refnum<class "Main.lvclass">)
            n237 = call "Fire Private Event.vi"("error in (no error)"=w591, "vData"=w587, "PrivAsync"=PrivateAsynEv_Main--enum."PrivMain.SetUnsetAlarm&ESRBLine", "Main in"=w593) -> ("error out"=w592:errorcluster)  [unwired: 6 in, 1 out]
          }
          event "reset averaging": Value Change {
            n238 = event-data() -> ()  [unwired: 1 in, 1 out]
            n239 = Unbundle By Name(w600) -> ("Self Reference"=w599:refnum<class "Main.lvclass">)
            n240 = call "Fire Private Event.vi"("error in (no error)"=w597, "PrivAsync"=PrivateAsynEv_Main--enum."PrivMain.ResetAveraging", "Main in"=w599) -> ("error out"=w598:errorcluster)  [unwired: 7 in, 1 out]
          }
          event User Event {
            n241 = event-data() -> ("notifier out"=w605:refnum<notifier>)  [unwired: 1 in]
            n242 = Bundle By Name(cluster=w607, "process sync"=w605) -> (w606:T12)
            n243 = call <vilib>:"Add State(s) to Queue__JKI_lib_State_Machine.vi"("State(s) in Front (\"\")"="Macro: Exit", "State(s) in (\"\")"=w604) -> ("States Out"=w603:string)  [unwired: 13 in]
          }
          event User Event {
            n244 = event-data() -> ("CmdMsg"=w614:string, "vData"=w618:variant)  [unwired: 1 in, 1 out]
            n245 = Unbundle By Name(w609) -> ("Self Reference"=w610:refnum<class "Main.lvclass">)
            n246 = call "get async cmd.vi"("error in (no error)"=w616, "Cmd String in"=w614) -> ("error out"=w615:errorcluster, "AsyncCmd"=w613:T62)  [unwired: 8 in]
            n247 = case shown="\"Main.StartProcessing\"" w613 {
              tunnel: w618 -> [_ w633 w644 w657]
              tunnel: w615 -> [w626 w632 w643 w656]
              tunnel: [w625 w631 w642 w655] -> w617
              tunnel: [_ "" "" "UI: Initialize InverterLUT List"] -> w612
              tunnel: w609 -> [w621 w629 w640 w654]
              tunnel: [w621 w628 w639 w653] -> w611
              tunnel: w610 -> [_ _ _ _]
              tunnel: w609 -> [_ _ _ _]
              frame Default {
                n248 = call <vilib>:"Build Error Cluster_ModKT .vi"("Prepend String (\"\")"="Invalid Async Cmd" ("Prepend String (\"\")"), "code"=42, "error? (F)"=TRUE, "error in (no error)"=w626) -> ("error out"=w625:errorcluster)  [unwired: 3 in, 1 out]
              }
              frame "Main.StartProcessing" {
                n249 = disable-structure shown="Disabled" {
                  disable-tunnel: w633 -> [w636 _]
                  disable-tunnel: w632 -> [w635 w637]
                  disable-tunnel: [w634 w637] -> w631
                  frame Disabled {
                    n250 = Variant To Data(error in=w635, Variant=w636) -> (error out=w634:errorcluster)  [unwired: 1 in, 1 out]
                  }
                  frame Enabled {
                  }
                }
                n251 = Bundle By Name(cluster=w629, "vData"=variant) -> (w628:T12)
              }
              frame "Main.StopProcessing" {
                n252 = disable-structure shown="Disabled" {
                  disable-tunnel: w644 -> [w647 _]
                  disable-tunnel: w643 -> [w646 w648]
                  disable-tunnel: [w645 w648] -> w642
                  frame Disabled {
                    n253 = Variant To Data(error in=w646, Variant=w647) -> (error out=w645:errorcluster)  [unwired: 1 in, 1 out]
                  }
                  frame Enabled {
                  }
                }
                n254 = Bundle By Name(cluster=w640, "vData"=variant) -> (w639:T12)
              }
              frame "Main.RefreshInverterList" {
                n255 = disable-structure shown="Disabled" {
                  disable-tunnel: w657 -> [w660 _]
                  disable-tunnel: w656 -> [w659 w661]
                  disable-tunnel: [w658 w661] -> w655
                  frame Disabled {
                    n256 = Variant To Data(error in=w659, Variant=w660) -> (error out=w658:errorcluster)  [unwired: 1 in, 1 out]
                  }
                  frame Enabled {
                  }
                }
                n257 = property on="Trigger SelectInverter Event" class="Bool (strict)"() -> ("Value"=w650:bool)  [unwired: 2 in, 2 out]
                n258 = Not(x=w650) -> (.not. x?=w649:bool)
                n259 = property on="Trigger SelectInverter Event" class="Bool (strict)"("Val(Sgnl)"=w649) -> ()  [unwired: 2 in, 2 out]
                n260 = Bundle By Name(cluster=w654, "vData"=variant) -> (w653:T12)
              }
            }
            n261 = call <vilib>:"Add State(s) to Queue__JKI_lib_State_Machine.vi"("State(s) in Front (\"\")"=w612, "State(s) in (\"\")"=w620) -> ("States Out"=w619:string)  [unwired: 13 in]
          }
          event User Event {
            n262 = event-data() -> ("NEW State"=w667:T63)  [unwired: 1 in, 6 out]
            n263 = Unbundle By Name(w667) -> ("DAQState"=w666:T30)
            n264 = Equal?(x=w666, y=DAQState--enum."Running" ("DAQState")) -> (x = y?=w662:bool)
            "DAQEnabled" <- w662
            "DAQ Running" <- w662
            n265 = Bundle By Name(cluster=w663, "DAQEnabled"=w662) -> (w664:T12)
          }
          event User Event {
            w671 = LogState--enum."Running"  # LogState
            n266 = event-data() -> ("NEW State"=w675:T65)  [unwired: 1 in, 6 out]
            n267 = Unbundle By Name(w675) -> ("LogState"=w674:T64)
            n268 = Equal?(x=w674, y=w671) -> (x = y?=w670:bool)
            "LogEnabled" <- w670
            n269 = Bundle By Name(cluster=w672, "LoggingEnabled"=w670) -> (w673:T12)
          }
          event User Event {
            w679 = TDMSState--enum."Running"  # TDMSState
            n270 = event-data() -> ("NEW State"=w683:T67)  [unwired: 1 in, 6 out]
            n271 = Unbundle By Name(w683) -> ("TDMSState"=w682:T66)
            n272 = Equal?(x=w682, y=w679) -> (x = y?=w678:bool)
            "TDMSEnabled" <- w678
            n273 = Bundle By Name(cluster=w680, "TDMS Enabled"=w678) -> (w681:T12)
          }
          event User Event {
            n274 = event-data() -> ("NEW ProcessingState"=w692:T10)  [unwired: 1 in]
            n275 = Unbundle By Name(w696) -> ("SMQ"=w691:refnum<queue>)
            n276 = Equal?(x=w692, y=ProcessingState--enum."Running") -> (x = y?=→"Processing":bool)
            n277 = Bundle By Name(cluster=w696, "ProcessingState"=w692) -> (w697:T12)
            n278 = call <vilib>:"Add State to Queue with vData.vi"("queue in"=w691, "state in"="Action: UpdateSMData >> ProcessingState", "vData (\"\")"=w692, "error in"=w693) -> ("error out"=w694:errorcluster)  [unwired: 8 in, 3 out]
            n279 = property on="Equivalent Series Resistance (ESR)" class="WFChart (strict)"("YScale.FormatString"="%#_g" ("Y Scale.Format String"), "YScale.Minimum"=0.0 ("Y Scale.Range:Minimum"), "YScale.Maximum"=0.1 ("Y Scale.Range:Maximum"), "History Data"=T31 []) -> ()  [unwired: 2 in, 2 out]
          }
        }
      }
      frame "---------- Core ----------" {
        n280 = call <vilib>:"Add State(s) to Queue__JKI_lib_State_Machine.vi"("State(s) in (\"\")"=w704) -> ("States Out"=w703:string)  [unwired: 14 in]
      }
      frame "Initialize Core Data" {
        # "originally closed?"
        # "exe?"
        n281 = property class="VI"() -> ("Front Panel.Open"=w713:bool)  [unwired: 2 in, 2 out]
        n282 = property class="App"() -> ("App.Kind"=w712:T32)  [unwired: 2 in, 2 out]
        n283 = control-ref of="Current VI Reference"() -> (w706:refnum<vi>)
        n284 = Not(x=w713) -> (.not. x?=w710:bool)
        n285 = Equal?(x=w712, y=T32."Run Time System" ("Application:Kind")) -> (x = y?=w709:bool)
        n286 = Or(x=w710, y=w709) -> (x .or. y?=w707:bool)
        n287 = Bundle By Name(cluster=w708, "Core.Current VI Reference"=w706, "Core.Close Panel on Exit?"=w707) -> (w715:T12)
        n288 = call <vilib>:"Add State(s) to Queue__JKI_lib_State_Machine.vi"("State(s) in (\"\")"=w717) -> ("States Out"=w716:string)  [unwired: 14 in]
      }
      frame "Process Sync" {
        n289 = Unbundle By Name(w722) -> ("process sync"=w721:refnum<notifier>)
        n290 = Send Notification(notification=TRUE, notifier=w721, error in (no error)=w719) -> (error out=w718:errorcluster)  [unwired: 1 out]
        n291 = call <vilib>:"Add State(s) to Queue__JKI_lib_State_Machine.vi"("State(s) in (\"\")"=w725) -> ("States Out"=w724:string)  [unwired: 14 in]
      }
      frame "DE_Register" {
        n292 = Unbundle By Name(w735) -> ("Public Events"=w734:T15, "Dependency.DAQ"=w733:refnum<class "DAQ_Engine.lvclass">, "Dependency.Log_Engine"=w731:refnum<class "Log_Engine.lvclass">)
        n293 = property class="DAQ_Engine.lvclass"(reference=w733, error in=w726) -> (error out=w728:errorcluster, "Accessors:PublicEvents*"=w732:T68)  [unwired: 1 out]
        n294 = property class="Log_Engine.lvclass"(reference=w731, error in=w726) -> (error out=w729:errorcluster, "Accessors:PublicEvents*"=w730:T69)  [unwired: 1 out]
        n295 = Merge Errors(w728, w729) -> (w727:errorcluster)
        n296 = register-events(error in=w727, w734, w732, w730) -> (reference out=w737:refnum<event-registration>, error out=w736:errorcluster)  [unwired: 1 in]
      }
      frame "DE_Unregister" {
        n297 = Unregister For Events(event registration refnum=w740, error in=w739) -> ()  [unwired: 1 out]
      }
      frame "---------- Data ----------" {
        n298 = call <vilib>:"Add State(s) to Queue__JKI_lib_State_Machine.vi"("State(s) in (\"\")"=w747) -> ("States Out"=w746:string)  [unwired: 14 in]
      }
      frame "Data: CreateCtrlRefs" {
        (unwired) "CtrlLabel-IOName Config - TS.xml" ("name or relative path")
        # "#TODO: finish implementation"
        n299 = Unbundle By Name(w749) -> ()  [unwired: 1 out]
        n300 = Unbundle By Name(w749) -> ("Application"=w748:refnum<class "Application.lvclass">)
        n301 = call <userlib>:"Wait (ms)__ogtk.vi"("error in (no error)"=w756, "milliseconds to wait"=u32 4000) -> ("error out"=w751:errorcluster)  [unwired: 8 in, 1 out]
        n302 = call "FG - App Class Ref.vi"("Application in"=w748, "error in (no error)"=w751, "action (Get)"=TD_GetSet_ActionSelect--enum."Set") -> ("Application out"=w753:refnum<class "Application.lvclass">, "error out"=w752:errorcluster)  [unwired: 6 in]
        n303 = call "Generate Async Msg Event.vi"("error in (no error)"=w752, "AsyncMsg"=AsynMsg_Application--enum."Application.AppClassReference", "Application in"=w753) -> ("error out"=w750:errorcluster)  [unwired: 7 in, 1 out]
        n304 = call <vilib>:"Add State(s) to Queue__JKI_lib_State_Machine.vi"("State(s) in (\"\")"=w760) -> ("States Out"=w759:string)  [unwired: 14 in]
      }
      frame "Data: Initialize" {
        w771 = FALSE ("DAQ Running")
        w786 = T70 {"Current VI Reference"=refnum, "Close Panel on Exit?"=FALSE}  # Core
        # "#TODO: add more items for\ninitialization here."
        n305 = Unbundle By Name(w780) -> ("DAQEnabled"=w779:bool, "LoggingEnabled"=w778:bool, "TDMS Enabled"=w777:bool, "Settings.Signal scaling"=w776:T2[], "Settings.ESR scaling"=w769:T8[], "Settings.num readings to average"=w775:i32[], "Settings.ESR alarm threshhold (%)"=w774:i32[], "Settings.UseDummyVrms"=w773:bool, "Settings.Dummy Vrms"=w772:dbl, "Dependency.DAQ"=w768:refnum<class "DAQ_Engine.lvclass">)
        n306 = property class="DAQ_Engine.lvclass"(reference=w768) -> ("Accessors:MeasSettings*"=w767:T5)  [unwired: 1 in, 2 out]
        n307 = Unbundle By Name(w780) -> ("StatusMsg Ref"=w782:refnum<vi>)
        n308 = Index Array(array=w775) -> (element=w762:i32)  [unwired: 1 in]
        n309 = Unbundle By Name(w767) -> ("Data Rate 9775"=w766:dbl, "Data Rate 9215"=w765:dbl, "Samples RMS 9215"=w764:u32, "Samples RMS 9775"=w763:u32)
        n310 = Index Array(array=w774) -> (element=w761:i32)  [unwired: 1 in]
        n311 = local write "Settings.Signal scaling"(w776) -> ()
        n312 = call <vilib>:"format status message v2.vi"("status msg"="Running Main UI", "Str Refnum"=w782) -> ()  [unwired: 5 in, 5 out]
        n313 = local write "ESR scaling"(w769) -> ()
        n314 = local write "# readings to average"(w762) -> ()
        n315 = local write "ESR alarm threshhold (%)"(w761) -> ()
        n316 = local write "UseDummyVrms"(w773) -> ()
        n317 = local write "DAQEnabled"(w779) -> ()
        n318 = local write "LogEnabled"(w778) -> ()
        n319 = local write "TDMSEnabled"(w777) -> ()
        n320 = local write "Dummy Vrms"(w772) -> ()
        n321 = local write "Data Rate 9215 (S/s)"(w765) -> ()
        n322 = local write "Data Rate 9775(S/s)"(w766) -> ()
        n323 = local write "Samples RMS 9215"(w764) -> ()
        n324 = local write "Samples RMS 9775"(w763) -> ()
        n325 = Current VI's Menubar() -> (w783:refnum<k9>)
        n326 = Bundle By Name(cluster=w780, "Core"=w786, "MenuRef"=w783) -> (w785:T12)
        n327 = local write "DAQ Running"(w771) -> ()
        n328 = local write "Processing"(w771) -> ()
        n329 = local write "Inverter ID"("") -> ()
        n330 = call <vilib>:"Add State(s) to Queue__JKI_lib_State_Machine.vi"("State(s) in (\"\")"=w789) -> ("States Out"=w788:string)  [unwired: 14 in]
      }
      frame "Data: Cleanup" {
        n331 = Unbundle By Name(w791) -> ("Core.Current VI Reference"=w794:refnum<vi>)
        n332 = Close Reference(reference=w794, error in (no error)=w793) -> (error out=w792:errorcluster)
        n333 = call <vilib>:"Add State(s) to Queue__JKI_lib_State_Machine.vi"("State(s) in (\"\")"=w796) -> ("States Out"=w795:string)  [unwired: 14 in]
      }
      frame "---------- UI ----------" {
        n334 = call <vilib>:"Add State(s) to Queue__JKI_lib_State_Machine.vi"("State(s) in (\"\")"=w801) -> ("States Out"=w800:string)  [unwired: 14 in]
      }
      frame "UI: Launch ESR Gain&Offset Explorer" {
        n335 = vi-ref "Control UI - Gain and Offset Exploration.vi"() -> (w806:refnum<vi>)
        n336 = Unbundle By Name(w810) -> ("Self Reference"=w809:refnum<class "Main.lvclass">)
        n337 = control-ref of="ESR scaling"() -> (w802:refnum<vi>)
        n338 = property class="VI"(reference=w806) -> ("Path"=w805:path)  [unwired: 1 in, 2 out]
        n339 = Open VI Reference(type specifier VI Refnum (for type only)=refnum<vi> refnum, vi path=w805, options=128, error in (no error)=w808) -> (vi reference=w803:refnum<vi>, error out=w807:errorcluster)  [unwired: 2 in]
        n340 = call-by-ref "Start Asynchronous Call"(reference=w803, error in=w807, "ESR scaling ref"=w802, "Main Ref"=w809) -> (reference out=w813:refnum<vi>, error out=w812:errorcluster)  [unwired: 10 in]
        n341 = Close Reference(reference=w813, error in (no error)=w812) -> (error out=w811:errorcluster)
        n342 = call <vilib>:"Add State(s) to Queue__JKI_lib_State_Machine.vi"("State(s) in (\"\")"=w817) -> ("States Out"=w816:string)  [unwired: 14 in]
      }
      frame "UI: Initialize InverterLUT List" {
        n343 = Unbundle By Name(w823) -> ("Self Reference"=w829:refnum<class "Main.lvclass">)
        n344 = property class="Main.lvclass"(reference=w829, error in=w825) -> (error out=w826:errorcluster, "Accessors:InvLUTDict*"=w828:T18, "Accessors:CurrInverter*"=w827:T37[])  [unwired: 1 out]
        n345 = for {
          tunnel: w827 -> [w837] mode=indexing
          tunnel: [w836] -> w822 mode=indexing
          n346 = Unbundle By Name(w837) -> ("name"=w836:string)
        }
        n347 = local write "Selected Inverter"(w822) -> ()
        n348 = call <vilib>:"Get ALL Dynamic CVT Data.vi"("error in (no error)"=w826, "dCVT DVR"=w828) -> ("error out"=w818:errorcluster, "NameArray"=w820:string[], "dCVT DVR out"=w819:T18)  [unwired: 6 in, 1 out]
        n349 = for {
          tunnel: w822 -> [w835] mode=indexing
          tunnel: [w834] -> w821 mode=indexing
          tunnel: w820 -> [w833]
          n350 = Search 1D Array(1D array=w833, element=w835) -> (index of element=w834:i32)  [unwired: 1 in]
        }
        n351 = case shown="No Error" w818 {
          frame No Error {
            n352 = local write "InvSelLED"(TRUE ("InvSelLED")) -> ()
          }
          frame Error {
          }
        }
        n353 = Bundle By Name(cluster=w823, "InverterLUT Dict"=w819, "InverterNames[]"=w820) -> (w824:T12)
        n354 = property on="Inverter List" class="LstBox (strict)"("Item Names"=w820) -> ()  [unwired: 2 in, 2 out]
        n355 = local write "Inverter List"(w821) -> ()
        n356 = call <vilib>:"Add State(s) to Queue__JKI_lib_State_Machine.vi"("State(s) in (\"\")"=w832) -> ("States Out"=w831:string)  [unwired: 14 in]
      }
      frame "UI: Show About Dialog" {
        n357 = Unbundle By Name(w843) -> ("Core.Current VI Reference"=w842:refnum<vi>)
        n358 = global read "GBL System.vi" "AppVersion"() -> (w841:string)
        n359 = call "Call About Dialog.vi"("error in (no error)"=w839, "AppVer"=w841, "Main UI Ref"=w842) -> ("error out"=w840:errorcluster)  [unwired: 8 in]
        n360 = call <vilib>:"Add State(s) to Queue__JKI_lib_State_Machine.vi"("State(s) in (\"\")"=w846) -> ("States Out"=w845:string)  [unwired: 14 in]
      }
      frame "UI: Launch TDMS Viewer" {
        n361 = Unbundle By Name(w849) -> ("TDMS Enabled"=w850:bool)
        n362 = case shown="True" w850 {
          tunnel: "Do Not Open TDMS File While System is Writing to File." ("message") -> [_ w872]
          tunnel: [T34."Left Button" ("Which Button?") w868] -> w852
          frame False {
          }
          frame True {
            n363 = call <vilib>:"Three Button Dialog.vi"("Window Title (\"\")"="CAUTION" ("Window Title (\"\")"), "Center Button Text (\"No\")"="", "Left Button Text (\"Yes\")"="OK", "message"=w872) -> ("Which Button?"=w868:T34)  [unwired: 7 in]
          }
        }
        n364 = case shown="Default" w852 {
          tunnel: w847 -> [w865 w866]
          tunnel: [w864 w866] -> w848
          frame Default {
            n365 = vi-ref "Launch TDMS File Viewer.vi"() -> (w856:refnum<vi>)
            n366 = property class="VI"(reference=w856) -> ("Path"=w857:path)  [unwired: 1 in, 2 out]
            n367 = Open VI Reference(type specifier VI Refnum (for type only)=refnum<vi> refnum, vi path=w857, options=128, error in (no error)=w865) -> (vi reference=w863:refnum<vi>, error out=w860:errorcluster)  [unwired: 2 in]
            n368 = call-by-ref "Start Asynchronous Call"(reference=w863, error in=w860) -> (reference out=w859:refnum<vi>, error out=w858:errorcluster)  [unwired: 12 in]
            n369 = Close Reference(reference=w859, error in (no error)=w858) -> (error out=w864:errorcluster)
          }
          frame "Right Button" {
          }
        }
        n370 = call <vilib>:"Add State(s) to Queue__JKI_lib_State_Machine.vi"("State(s) in (\"\")"=w855) -> ("States Out"=w854:string)  [unwired: 14 in]
      }
      frame "UI: Initialize2" {
        w876 = FALSE
        w879 = FALSE
        n371 = Unbundle By Name(w873) -> ()  [unwired: 1 out]
        n372 = local write "MainPanelTab"(T6."ESRData" ("MainPanelTab")) -> ()
        n373 = local write "DataPg_button"(w879) -> ()
        n374 = local write "Page2Pg_button"(w879) -> ()
        n375 = local write "ConfigPg_button"(w879) -> ()
        n376 = local write "SettingsPg_button"(TRUE) -> ()
        n377 = local write "LeftPanelTab"(T1."Settings" ("LeftPanelTab")) -> ()
        n378 = local write "Sel_ESR_Data"(TRUE) -> ()
        n379 = local write "Sel_TimeSeries_Data"(w876) -> ()
        n380 = local write "Sel_PowerFactor_Data"(w876) -> ()
        n381 = call <vilib>:"Add State(s) to Queue__JKI_lib_State_Machine.vi"("State(s) in (\"\")"=w883) -> ("States Out"=w882:string)  [unwired: 14 in]
      }
      frame "UI: Initialize" {
        w884 = FALSE
        # "#TODO: add Remote error handling menu items"
        n382 = Unbundle By Name(w885) -> ("Core.Current VI Reference"=w890:refnum<vi>)
        n383 = call <userlib>:"Fit VI window to Largest Dec__ogtk.vi"("error in (no error)"=w892, "VI Ref (calling VI)"=w890) -> ("error out"=w891:errorcluster, "dup VI Ref"=w889:refnum<vi>)  [unwired: 4 in]
        n384 = global read "GBL System.vi" "AppVersion"() -> (w888:string)
        n385 = property class="VI"(reference=w889, "Front Panel.Title"=w888) -> (reference out=w887:refnum<vi>)  [unwired: 1 in, 1 out]
        n386 = local write "TitleBar AppVerText"(w888) -> ()
        n387 = Bundle By Name(cluster=w885, "MenuBarShown?"=w884) -> (w886:T12)
        n388 = property class="VI"(reference=w887, "Front Panel.ShowMenuBar"=w884) -> ()  [unwired: 1 in, 2 out]
        n389 = call <vilib>:"Add State(s) to Queue__JKI_lib_State_Machine.vi"("State(s) in (\"\")"=w895) -> ("States Out"=w894:string)  [unwired: 14 in]
      }
      frame "UI: Cursor Set" {
        # "Argument"
        n390 = case shown="\"Idle\", Default" w897 {
          tunnel: w899 -> [w904 w906]
          tunnel: [w903 w905] -> w898
          frame "Idle", Default {
            n391 = call <vilib>:"Unset Busy.vi"("error in (no error)"=w904) -> ("error out"=w903:errorcluster)  [unwired: 10 in]
          }
          frame "Busy" {
            n392 = call <vilib>:"Set Busy.vi"("error in (no error)"=w906) -> ("error out"=w905:errorcluster)  [unwired: 9 in, 1 out]
          }
        }
        n393 = call <vilib>:"Add State(s) to Queue__JKI_lib_State_Machine.vi"("State(s) in (\"\")"=w902) -> ("States Out"=w901:string)  [unwired: 14 in]
      }
      frame "UI: Front Panel State" {
        # "Argument"
        n394 = Unbundle By Name(w911) -> ("Core.Current VI Reference"=w914:refnum<vi>)
        n395 = Unbundle By Name(w911) -> ("Splash VI Ref"=w910:refnum<vi>, "Splash StatusRef"=w907:refnum<vi>, "StatusMsg Ref"=w908:refnum<vi>)
        n396 = case shown="\"Close\"" w913 {
          tunnel: w916 -> [w922 w941]
          tunnel: [w924 w933] -> w915
          tunnel: w914 -> [w923 w939]
          tunnel: w910 -> [_ w936]
          tunnel: "Quitting  IHS\nPlease Wait . . ." ("FP Msg") -> [_ w935]
          tunnel: w907 -> [_ w931]
          tunnel: w908 -> [_ w932]
          frame "Open", Default {
            n397 = property class="VI"(reference=w923, error in=w922) -> (reference out=w920:refnum<vi>, error out=w921:errorcluster, "Front Panel.Open"=w919:bool)
            n398 = case shown="True" w919 {
              tunnel: [w927 w930] -> w924
              tunnel: w921 -> [w926 w930]
              tunnel: w920 -> [w925 _]
              frame False {
                n399 = invoke class="VI" method="FP.Open"(reference=w925, error in=w926, "Activate"=TRUE, "State"=T35."Standard") -> (error out=w927:errorcluster)  [unwired: 1 in, 4 out]
              }
              frame True {
              }
            }
          }
          frame "Close" {
            n400 = property class="VI"(reference=w939, error in=w941) -> (reference out=w938:refnum<vi>, error out=w940:errorcluster, "Front Panel.Open"=w937:bool)
            n401 = case shown="True" w937 {
              tunnel: [w962 w965] -> w934
              tunnel: w940 -> [w962 w964]
              tunnel: w938 -> [_ w963]
              frame False {
              }
              frame True {
                n402 = invoke class="VI" method="FP.Close"(reference=w963, error in=w964) -> (error out=w965:errorcluster)  [unwired: 1 in, 2 out]
              }
            }
            n403 = disable-structure shown="Disabled" {
              disable-tunnel: w936 -> [w957 _]
              disable-tunnel: w935 -> [w955 _]
              disable-tunnel: w934 -> [w953 w961]
              disable-tunnel: [w952 w961] -> w933
              disable-tunnel: w932 -> [w943 _]
              disable-tunnel: w931 -> [w942 _]
              frame Disabled {
                n404 = property class="Str"(reference=w943) -> (error out=w944:errorcluster, "Value"=w948:string)  [unwired: 1 in, 1 out]
                n405 = call "FG - StatusStrRef.vi"("StatusStr Ref in"=w942, "error in (no error)"=w944, "action (Get)"=TD_GetSet_ActionSelect--enum."Set") -> ("StatusStr Ref out"=w946:refnum<vi>, "error out"=w945:errorcluster)  [unwired: 6 in]
                n406 = call <userlib>:"Set Control Value {Variant}__ogtk.vi"("error in (no error)"=w953, "Control Name (\"\": use variant name)"="FP Msg", "Value"=w955, "VI Refnum"=w957) -> ("error out"=w954:errorcluster, "VI Refnum dup"=w958:refnum<vi>)  [unwired: 6 in]
                n407 = property class="Str"(reference=w946, error in=w945, "Value"=w948) -> (reference out=w949:refnum<vi>, error out=w950:errorcluster)
                n408 = property class="VI"(reference=w958, error in=w954, "FP.Behavior"=T36."Modal" ("Front Panel Window:Behavior"), "FP.State"=T35."Standard" ("Front Panel Window:State")) -> (error out=w952:errorcluster)  [unwired: 1 out]
                n409 = property class="Str"(reference=w949, error in=w950, "Text.Scroll Position"=u32 999999999) -> ()  [unwired: 2 out]
              }
              frame Enabled {
              }
            }
          }
        }
        n410 = call <vilib>:"Add State(s) to Queue__JKI_lib_State_Machine.vi"("State(s) in (\"\")"=w918) -> ("States Out"=w917:string)  [unwired: 14 in]
      }
      frame "---------- Macro ----------" {
        n411 = call <vilib>:"Add State(s) to Queue__JKI_lib_State_Machine.vi"("State(s) in (\"\")"=w970) -> ("States Out"=w969:string)  [unwired: 14 in]
      }
      frame "Macro: Initialize" {
        n412 = call <vilib>:"Add State(s) to Queue__JKI_lib_State_Machine.vi"("State(s) in Front (\"\")"=w971, "State(s) in (\"\")"=w976) -> ("States Out"=w975:string)  [unwired: 13 in]
      }
      frame "Macro: Exit" {
        n413 = Unbundle By Name(w992) -> ("Core.Close Panel on Exit?"=w991:bool, "LoggingEnabled"=w982:bool, "TDMS Enabled"=w984:bool, "DAQEnabled"=w983:bool)
        n414 = Compound Arithmetic op=OR(w982, w984, w983) -> (w980:bool)
        n415 = Select(t="Action: Stop Daq & Logging", s=w980, f="") -> (s? t:f=w977:string)
        n416 = call <vilib>:"Add State(s) to Queue__JKI_lib_State_Machine.vi"("State(s) in Front (\"\")"=w977, "State(s) in (\"\")"=w981) -> ("States Out"=w985:string)  [unwired: 13 in]
        n417 = Select(t="UI: Front Panel State >> Close", s=w991, f="") -> (s? t:f=w987:string)
        n418 = Format Into String(format string=w985, w987) -> (resulting string=w986:string)  [unwired: 2 in, 1 out]
        n419 = call <vilib>:"Add State(s) to Queue__JKI_lib_State_Machine.vi"("State(s) in Front (\"\")"=w986, "State(s) in (\"\")"=w995) -> ("States Out"=w994:string)  [unwired: 13 in]
      }
      frame "---------- Action ----------" {
        n420 = call <vilib>:"Add State(s) to Queue__JKI_lib_State_Machine.vi"("State(s) in (\"\")"=w1000) -> ("States Out"=w999:string)  [unwired: 14 in]
      }
      frame "Action: Open Inverter LUT DB Editor" {
        n421 = Unbundle By Name(w1012) -> ("Self Reference"=w1003:refnum<class "Main.lvclass">, "Core.Current VI Reference"=w1001:refnum<vi>)
        n422 = vi-ref "Inverter LUT UI.vi"() -> (w1007:refnum<vi>)
        n423 = property class="VI (strict)"(reference=w1007) -> (reference out=w1004:refnum<vi>, "Path"=w1006:path)  [unwired: 1 in, 1 out]
        n424 = Open VI Reference(type specifier VI Refnum (for type only)=w1004, vi path=w1006, options=128) -> (vi reference=w1005:refnum<vi>, error out=w1009:errorcluster)  [unwired: 3 in]
        n425 = call-by-ref "Start Asynchronous Call"(reference=w1005, error in=w1009, "Caller VI Refnum (Callee's Caller)"=w1001, "Main in"=w1003) -> (reference out=w1002:refnum<vi>, error out=w1010:errorcluster)  [unwired: 9 in, 1 out]
        n426 = Close Reference(reference=w1002, error in (no error)=w1010) -> (error out=w1011:errorcluster)
        n427 = call <userlib>:"Clear All Errors__ogtk.vi"("Error In"=w1011) -> ()  [unwired: 3 in, 1 out]
        n428 = call <vilib>:"Add State(s) to Queue__JKI_lib_State_Machine.vi"("State(s) in (\"\")"=w1016) -> ("States Out"=w1015:string)  [unwired: 14 in]
      }
      frame "Action: View Inverter Param Values" {
        n429 = local read "Inverter List"() -> (w1028:i32[])
        n430 = Unbundle By Name(w1030) -> ("Core.Current VI Reference"=w1029:refnum<vi>)
        n431 = Unbundle By Name(w1030) -> ("Self Reference"=w1031:refnum<class "Main.lvclass">)
        n432 = property on="Inverter List" class="LstBox (strict)"() -> ("Item Names"=w1027:string[])  [unwired: 2 in, 2 out]
        n433 = Index Array(array=w1028) -> (element=w1017:i32)  [unwired: 1 in]
        n434 = Index Array(array=w1027, index=w1017) -> (element=w1025:string)
        n435 = property class="Main.lvclass"(reference=w1031) -> (error out=w1024:errorcluster, "Accessors:InvLUTDict*"=w1026:T18)  [unwired: 1 in, 1 out]
        n436 = vi-ref "View Selected Inverter Parameter Values.vi"() -> (w1032:refnum<vi>)
        n437 = property class="VI (strict)"(reference=w1032) -> (reference out=w1034:refnum<vi>, "Path"=w1036:path)  [unwired: 1 in, 1 out]
        n438 = Open VI Reference(type specifier VI Refnum (for type only)=w1034, vi path=w1036, options=128) -> (vi reference=w1035:refnum<vi>, error out=w1038:errorcluster)  [unwired: 3 in]
        n439 = call <vilib>:"Get Dynamic CVT Data.vi"("error in (no error)"=w1024, "DataName"=w1025, "dCVT DVR"=w1026) -> ("error out"=w1022:errorcluster, "value"=w1023:variant)  [unwired: 5 in, 2 out]
        n440 = Variant To Data(error in=w1022, type=T37 {"name"="", "last updated"=timestamp(0 s since 1904-01-01), "type"="", "inverter Info"={"manufacturer"="", "model"="", "product"="", "serial"="", "power class"="", "year manf"=""}, "gain range"={"gain max"=0.0, "gain min"=0.0, "gain increment"=0.0}, "offset range"={"offset max"=0.0, "offset min"=0.0, "offset increment"=0.0}, "gain actual"=0.0, "offset actual"=0.0, "power level"=0.0, "minimum current"=0.0, "resistance single phase"=0.0, "resistance 3 phase"=0.0, "set flag"=0} ("Inverter v2"), Variant=w1023) -> (data=w1020:T37, error out=w1018:errorcluster)
        n441 = case shown="No Error" w1018 {
          tunnel: [w1050 w1052] -> w1039
          tunnel: w1038 -> [w1049 w1052]
          tunnel: w1035 -> [w1048 w1051]
          tunnel: [w1047 w1051] -> w1033
          tunnel: w1029 -> [w1046 _]
          tunnel: w1020 -> [w1045 _]
          frame No Error {
            n442 = call-by-ref "Start Asynchronous Call"(reference=w1048, error in=w1049, "Caller VI Refnum (Callee's Caller)"=w1046, "Inverter v2"=w1045) -> (reference out=w1047:refnum<vi>, error out=w1050:errorcluster)  [unwired: 10 in]
          }
          frame Error {
          }
        }
        n443 = Merge Errors(w1018, w1042) -> (w1019:errorcluster)
        n444 = Close Reference(reference=w1033, error in (no error)=w1039) -> (error out=w1040:errorcluster)
        n445 = call <userlib>:"Clear All Errors__ogtk.vi"("Error In"=w1040) -> ()  [unwired: 3 in, 1 out]
        n446 = call <vilib>:"Add State(s) to Queue__JKI_lib_State_Machine.vi"("State(s) in (\"\")"=w1044) -> ("States Out"=w1043:string)  [unwired: 14 in]
      }
      frame "Action: Stop Daq & Logging" {
        n447 = Unbundle By Name(w1073) -> ("TDMS Enabled"=w1069:bool, "Dependency.Log_Engine"=w1070:refnum<class "Log_Engine.lvclass">, "LoggingEnabled"=w1060:bool, "Dependency.DAQ"=w1072:refnum<class "DAQ_Engine.lvclass">, "DAQEnabled"=w1071:bool)
        n448 = Not(x=w1069) -> (.not. x?=w1068:bool)
        n449 = call "CMD StopLog.vi"("error in (no error)"=w1053, "bypass (F)"=w1068, "Log_Engine in"=w1070) -> ("error out"=w1055:errorcluster, "Log_Engine out"=w1063:refnum<class "Log_Engine.lvclass">)  [unwired: 7 in]
        n450 = Not(x=w1060) -> (.not. x?=w1059:bool)
        n451 = Select(t=u32 0, s=w1068, f=u32 2000 ("milliseconds to wait")) -> (s? t:f=w1065:u32)
        n452 = call <userlib>:"Wait (ms)__ogtk.vi"("error in (no error)"=w1055, "milliseconds to wait"=w1065) -> ("error out"=w1064:errorcluster)  [unwired: 8 in, 1 out]
        n453 = Select(t=u32 0, s=w1059, f=u32 1000 ("milliseconds to wait")) -> (s? t:f=w1057:u32)
        n454 = call "CMD StopESRLog.vi"("error in (no error)"=w1064, "bypass (F)"=w1059, "Log_Engine in"=w1063) -> ("error out"=w1058:errorcluster)  [unwired: 7 in, 1 out]
        n455 = call <userlib>:"Wait (ms)__ogtk.vi"("error in (no error)"=w1058, "milliseconds to wait"=w1057) -> ("error out"=w1056:errorcluster)  [unwired: 8 in, 1 out]
        n456 = case shown="True" w1071 {
          tunnel: w1072 -> [_ w1083]
          tunnel: w1056 -> [w1077 w1081]
          tunnel: [w1077 w1078] -> w1054
          frame False {
          }
          frame True {
            n457 = call "CMD StartStopDAQ.vi"("error in (no error)"=w1081, "DAQEnable"=FALSE, "DAQ_Engine in"=w1083) -> ("error out"=w1080:errorcluster)  [unwired: 7 in, 1 out]
            n458 = call <userlib>:"Wait (ms)__ogtk.vi"("error in (no error)"=w1080, "milliseconds to wait"=u32 1000) -> ("error out"=w1078:errorcluster)  [unwired: 8 in, 1 out]
          }
        }
        n459 = call <vilib>:"Add State(s) to Queue__JKI_lib_State_Machine.vi"("State(s) in (\"\")"=w1076) -> ("States Out"=w1075:string)  [unwired: 14 in]
      }
      frame "Action: SendParamsToProcess" {
        # "This should work, but has not been tested yet"
        n460 = local read "Settings.Signal scaling"() -> (w1094:T2[])
        n461 = local read "UseDummyVrms"() -> (w1091:bool)
        n462 = Unbundle By Name(w1096) -> ("Self Reference"=w1095:refnum<class "Main.lvclass">)
        n463 = local read "Dummy Vrms"() -> (w1092:dbl)
        n464 = local read "ESR scaling"() -> (w1084:T8[])
        n465 = To Variant(anything=w1094) -> (Variant=w1093:variant)
        n466 = To Variant(anything=w1091) -> (Variant=w1090:variant)
        n467 = To Variant(anything=w1092) -> (Variant=w1089:variant)
        n468 = To Variant(anything=w1084) -> (Variant=w1088:variant)
        n469 = Build Array(w1093, w1090, w1089, w1088) -> (w1087:variant[])
        n470 = for {
          tunnel: w1095 -> [w1105]
          shift-right: [w1103] -> w1086
          shift-left: w1085 -> [w1101]
          tunnel: w1087 -> [w1100] mode=indexing
          n471 = call "Fire UpdateControlValue Event.vi"("error in (no error)"=w1101, "vData"=w1100, "Main in"=w1105) -> ("error out"=w1104:errorcluster)  [unwired: 7 in, 1 out]
          n472 = call <userlib>:"Wait (ms)__ogtk.vi"("error in (no error)"=w1104, "milliseconds to wait"=u32 500) -> ("error out"=w1103:errorcluster)  [unwired: 8 in, 1 out]
        }
        n473 = call <vilib>:"Add State(s) to Queue__JKI_lib_State_Machine.vi"("State(s) in (\"\")"=w1099) -> ("States Out"=w1098:string)  [unwired: 14 in]
      }
      frame "Action: Shutdown System" {
        # "delay to ensure shutdown status messages\ncan be read in the UI"
        n474 = Unbundle By Name(w1113) -> ("StatusMsg Ref"=w1110:refnum<vi>, "AppTerminateEv"=w1112:refnum<user-event>)
        n475 = call "Fire StopProcess Event.vi"("error in (no error)"=w1106, "Event in"=w1112) -> ("error out"=w1107:errorcluster)  [unwired: 6 in, 3 out]
        n476 = call <userlib>:"Wait (ms)__ogtk.vi"("error in (no error)"=w1107, "milliseconds to wait"=u32 4500) -> ("error out"=w1108:errorcluster)  [unwired: 8 in, 1 out]
        n477 = call <vilib>:"format status message v2.vi"("status msg"="Shutting down Main UI", "Str Refnum"=w1110) -> ()  [unwired: 5 in, 5 out]
        n478 = disable-structure shown="Disabled" {
          frame Disabled {
            n479 = Generate User Event(event data cluster=refnum<notifier> refnum ("event data")) -> ()  [unwired: 3 in, 2 out]
          }
          frame Enabled {
          }
        }
        n480 = call <vilib>:"Add State(s) to Queue__JKI_lib_State_Machine.vi"("State(s) in (\"\")"=w1116) -> ("States Out"=w1115:string)  [unwired: 14 in]
      }
      frame "Action: Wait" {
        n481 = Scan From String(format string="%d", input string=w1118, error in=w1120, default 1=u32 0) -> (error out=w1124:errorcluster, output 1=w1123:u32)  [unwired: 1 in, 2 out]
        n482 = call <userlib>:"Wait (ms)__ogtk.vi"("error in (no error)"=w1124, "milliseconds to wait"=w1123) -> ("error out"=w1119:errorcluster)  [unwired: 8 in, 1 out]
        n483 = call <vilib>:"Add State(s) to Queue__JKI_lib_State_Machine.vi"("State(s) in (\"\")"=w1128) -> ("States Out"=w1127:string)  [unwired: 14 in]
      }
      frame "Action: Terminate AsyncLoop" {
        n484 = Unbundle By Name(w1134) -> ("SMQ"=w1133:refnum<queue>)
        n485 = Flush Queue(queue=w1133) -> (queue out=w1132:refnum<queue>)  [unwired: 1 in, 2 out]
        n486 = call <vilib>:"Add State to Queue with vData.vi"("queue in"=w1132, "state in"="Macro: Exit", "error in"=w1130) -> ("error out"=w1129:errorcluster)  [unwired: 9 in, 3 out]
        n487 = call <vilib>:"Add State(s) to Queue__JKI_lib_State_Machine.vi"("State(s) in (\"\")"=w1137) -> ("States Out"=w1136:string)  [unwired: 14 in]
      }
    }
  }
  n488 = Merge Errors(w3, w2) -> ()  [unwired: 1 out]
